vi "WHD_VEten_0.1_BIDIREC_Pruebas.vi"() -> ()   [LabVIEW 2015]
uses:
  <vilib>/NI_Real-Time Target Support.lvlib
  <vilib>/rvi/interface/nirviReadWriteControl/nirviReadWriteControl.xnode
  <vilib>/rvi/interface/nirviMethod/nirviMethod.xnode
  <vilib>/rvi/interface/nirviOpenFPGA/nirviOpenFPGA.xnode
  <vilib>/rvi/interface/nirviCloseFPGA/nirviCloseFPGA.xnode
  <vilib>/real-time/NI_Real-Time Libraries.lvlib
  <vilib>/userdefined/High Color/nirio_resource_hc.ctl
  <vilib>/Utility/file.llb/Write To Spreadsheet File (string).vi
  AURA_Wheel/Json2Labv.lvlib
  AURA_Wheel/AuraWheelAPI/AuraWheel.lvlib
  <vilib>/LabVIEW Targets/FPGA/cRIO/shared/nicrio_ModuleControls/nicrio_cRIO-9234_DataRatesRing2.ctl
  <vilib>/real-time/rtutility.llb/RT Restart Target (Self).vi
  FPGA Bitfiles/W&RDEuskotren_FPGATarget_FPGA8awsBIdirecc_10D55B35.lvbitx
  <vilib>/FPGAPlugInAG/cRIO-9113/niLvFpga_Open_cRIO-9113.vi
  <vilib>/FPGAPlugInAG/cRIO-9113/niLvFpga_Run_cRIO-9113.vi
  NiFpgaLv.dll
  <vilib>/Utility/error.llb/Error Cluster From Error Code.vi
  <vilib>/rvi/errors/niLvFpgaAdjustHostInterfaceError.vi
  <vilib>/FPGAPlugInAG/cRIO-9113/niLvFpga_ConfigureFifo_cRIO-9113.vi
  <vilib>/rvi/errors/niLvFpgaMergeErrorWithErrorCode.vi
  <vilib>/FPGAPlugInAG/cRIO-9113/niLvFpga_StartFifo_cRIO-9113.vi
  <vilib>/FPGAPlugInAG/cRIO-9113/niLvFpga_ReadFifo_cRIO-9113.vi
  <vilib>/FPGAPlugInAG/cRIO-9113/niLvFpga_StopFifo_cRIO-9113.vi
  <vilib>/FPGAPlugInAG/cRIO-9113/niLvFpga_Reset_cRIO-9113.vi
  <vilib>/FPGAPlugInAG/cRIO-9113/niLvFpga_Close_cRIO-9113.vi
  <vilib>/RTwatchdog.llb/Watchdog expiration actions.ctl
panel:
  out "TAGs_AURAwheel":string[][](array[string])
  out "Plataformas?":bool
  out "Ejes_convoy":i32
  out "Nº Ejes":i32[](array[numeric])
  out "Nº UTs":i32
  out "it-read-LR6":i32[](array[numeric])
  out "it-LR6":i32
  out "RFID_LR6_Error":errorcluster
  out "TAGs HEX":string[](array[string])
  out "TAGs LR6":string[](array[string])
  in  "TAGs HEX 2":string[](array[string])
  out "Series_flota":string[](array[string])
  out "Tabla_flota":string[][](array[string])
  out "Puntos medios de las ventanas":dbl[][](array[numeric])
  in  "User":string
  in  "Índice de los archivos seleccionados":i32
  in  "Array":path[][](array[path])=[[path "c:/Trenes_prueba/0207_2013-09-24_19-09-42_0.bin", path "c:/Trenes_prueba/0096_2013-10-30_18-13-14_0.bin", path "c:/Trenes_prueba/0001_2013-06-05_13-06-23_0.bin"], [path "c:/Trenes_prueba/0207_2013-09-24_19-09-42_1.bin", path "c:/Trenes_prueba/0096_2013-10-30_18-13-14_1.bin", path "c:/Trenes_prueba/0001_2013-06-05_13-06-23_1.bin"], [path "c:/Trenes_prueba/0207_2013-09-24_19-09-42_2.bin", path "c:/Trenes_prueba/0096_2013-10-30_18-13-14_2.bin", path "c:/Trenes_prueba/0001_2013-06-05_13-06-23_2.bin"], [path "c:/Trenes_prueba/0207_2013-09-24_19-09-42_3.bin", path "c:/Trenes_prueba/0096_2013-10-30_18-13-14_3.bin", path "c:/Trenes_prueba/0001_2013-06-05_13-06-23_3.bin"], [path "c:/Trenes_prueba/0207_2013-09-24_19-09-42_4.bin", path "c:/Trenes_prueba/0096_2013-10-30_18-13-14_4.bin", path "c:/Trenes_prueba/0001_2013-06-05_13-06-23_4.bin"], [path "c:/Trenes_prueba/0207_2013-09-24_19-09-42_5.bin", path "c:/Trenes_prueba/0096_2013-10-30_18-13-14_5.bin", path "c:/Trenes_prueba/0001_2013-06-05_13-06-23_5.bin"], [path "c:/Trenes_prueba/0207_2013-09-24_19-09-42_6.bin", path "c:/Trenes_prueba/0096_2013-10-30_18-13-14_6.bin", path "c:/Trenes_prueba/0001_2013-06-05_13-06-23_6.bin"], [path "c:/Trenes_prueba/0207_2013-09-24_19-09-42_7.bin", path "c:/Trenes_prueba/0096_2013-10-30_18-13-14_7.bin", path "c:/Trenes_prueba/0001_2013-06-05_13-06-23_7.bin"], [path "c:/Trenes_prueba/0207_2013-09-24_19-09-42_8.bin", path "c:/Trenes_prueba/0096_2013-10-30_18-13-14_8.bin", path "c:/Trenes_prueba/0001_2013-06-05_13-06-23_8.bin"]]
  out "configuration file path":path=path "c:/Parametros.cfg"
  in  "IP synchr":string
  in  "Canal ccero?":bool
  in  "Digital?":bool=TRUE
  out "Numeric 3":i32
  out "data":cluster{"status":string}
  out "confRFID":path=path "c:/RFID/TAGS.csv"
  out "TAGS leidos":path=path "c:/RFID/TAGS.csv"
  in  "Use Aura?":bool
  in  "Parametros AuraWheel":string[](array[string])
  in  "Parámetros acelerómetros":dbl[](array[numeric])
  in  "Number of Samples":u32=2000
  in  "x*y":dbl[](array[numeric])=array[252000 elements]
  out "RFID_Error 2":errorcluster
  in  "milliseconds to wait":u32=180000
  in  "Adquirir continuado":bool
  in  "Tiempo de adquisicion":dbl=10.0
  in  "Adquirir":bool
  in  "Señal digital?":bool=TRUE
  out "Inductivo OK?":bool=TRUE
  out "Acelerómetros OK?":bool[](array[boolean])
  out "Fin":bool
  out "Contador":i32=1
  in  "expiration actions":T1={"reset"=TRUE, "occurrence"=FALSE, "trigger protocol"=enum."active high", "trigger line"=enum."none", "disable watchdog on VI exit"=TRUE}
  out "Path TEST":path=path "c:/TEST"
  out "Fallo fotocelula":bool
  out "Path_Borrar":path=path "c:/Trenes"
  out "Longitud de la unidad":dbl
  out "Bucle Espera":i32
  out "Aviso no detección":string
  out "Time to Acquire Block (ms)":i32
  out "Distancia de acelerómetros":dbl[](array[numeric])
  out "Block Size":u32
  out "Distancias generales":dbl[](array[numeric])
  in  "Reset del controlador":bool
  in  "Configuración":bool
  in  "Parar la aplicación":bool
  out "Acel 4":bool=TRUE
  out "Acel 3":bool=TRUE
  out "Acel 2":bool=TRUE
  out "Acel 1":bool=TRUE
  out "RFID":bool=TRUE
  out "date/time string":string
  out "Obstruido?":bool
  out "Tiempo":dbl
  out "Inicio pasada":timestamp
  out "Ultimo TEST":timestamp
  out "Fuente":bool=TRUE
  out "Estado":string
  in  "Number of Channels":u32=9
  out "RFID_ID":refnum<k5>
  out "DC OK":string
  out "Aviso temperatura":string
  in  "Tab Control":T2(tab)=enum."Parámetros"
  out "V (m/s)":dbl
  out "Temperatura (ºC)":dbl
  out "Max RMS Ruedas":dbl[][](array[numeric])
  in  "Hora de borrado":string
  out "result":bool
  out "TAGs":string[](array[string])
  out "Nombre de archivo":path[](array[path])
  out "Tiempo de paso (s)":dbl
  out "Tiempo extra de adquisición (s)":dbl
  out "Número de ejes detectados":i32
  out "Buffer Underflow":bool
  out "Buffer Overflow":bool
  out "Disco Duro Disponible (bytes)":i64
  out "created path":path
  out "Fallo sensores":string
  out "T fuera rango":bool
  in  "Frecuencia de muestreo (Hz)":dbl=25600.0
  in  "Escaneos de la FIFO por canal":u32=1000
  in  "Tiempo extra al detector de paso (s)":dbl=1.0
  in  "Filtro digital (ms)":u16=13
  in  "dt RMS":dbl=256.0
  in  "Time":T3 {"Segundo" min=0 max=60; "Minuto" min=0 max=60; "Hora" min=0 max=24}
  in  "Cambiar hora":bool
  in  "Date":T4={"Mes   "=1, "Día         "=1, "Año "=2010} {"Año" min=1900 max=3000 step=1; "Día" min=1 max=31 step=1; "Mes" min=1 max=12 step=1}
  in  "Cambiar Fecha":bool
  in  "Frecuencia de muestreo y módulo CRIO":T5=2 items=["51.200 kS/s (NI 9234)"=1, "25.600 kS/s (NI 9234)"=2, "17.067 kS/s (NI 9234)"=3, "12.800 kS/s (NI 9234)"=4, "10.240 kS/s (NI 9234)"=5, "8.533 kS/s (NI 9234)"=6, "7.314 kS/s (NI 9234)"=7, "6.400 kS/s (NI 9234)"=8, "5.689 kS/s (NI 9234)"=9, "5.120 kS/s (NI 9234)"=10, "4.654 kS/s (NI 9234)"=11, "4.267 kS/s (NI 9234)"=12, "3.938 kS/s (NI 9234)"=13, "3.657 kS/s (NI 9234)"=14, "3.413 kS/s (NI 9234)"=15, "3.200 kS/s (NI 9234)"=16, "3.012 kS/s (NI 9234)"=17, "2.845 kS/s (NI 9234)"=18, "2.695 kS/s (NI 9234)"=19, "2.560 kS/s (NI 9234)"=20, "2.438 kS/s (NI 9234)"=21, "2.328 kS/s (NI 9234)"=22, "2.226 kS/s (NI 9234)"=23, "2.133 kS/s (NI 9234)"=24, "2.048 kS/s (NI 9234)"=25, "1.969 kS/s (NI 9234)"=26, "1.896 kS/s (NI 9234)"=27, "1.829 kS/s (NI 9234)"=28, "1.765 kS/s (NI 9234)"=29, "1.707 kS/s (NI 9234)"=30, "1.652 kS/s (NI 9234)"=31]
  in  "Puerto RFID":u16=2189
  in  "IP RFID":string="192.168.106.99"
  in  "Offset_rueda":fxp<+/-,24,-4>=0.004999998956918716 format="%.27g"
  in  "Count(mSec)":u32=2
  in  "LR6 IP address":string="192.168.106.94"
  in  "Port LR6":u16=2001
  out "Direccion 0?":bool
  in  "Pruebas RFID 2":bool
  in  "Pruebas RFID 1":bool
  in  "Descargar":bool
  out "Parámetros":bool=TRUE
  out "Distacias y medidas de dispositivos":bool=TRUE
  out "RFID_Error":errorcluster
  out "error FPGA":errorcluster
  out "error manipulacion archivos":errorcluster
  out "Unidades y ejes":bool=TRUE
  out "RFID":bool=TRUE
  out "error AURA":errorcluster
  out "Response headers":string
  # "Funciona?"
  # "Inductivo"
  # "A4"
  # "A3"
  # "A1"
  # "A2"
  # "WRD_MEX\nWRD_ZAR"
  # "0 tagMexInit\n1 tagMexFin\n\n0 tag1\n1 tag2"
  # "Última detección de unidad"
  # "Error!!"
  # "Estado de la memoria"
  # "Espera"
  # "Adquisicion"
  # "Adquisicion"
  # "Procesado"
  # "Procesado"
  # "Procesado"
  # "Procesado"
  # "Procesado"
  # "Parámetros de muestreo"
  # "Parámetros de adquisición"
  # "Parámetros de procesado"
  # "Cambio Fecha y Hora"
  # "Descarga de planos y TEST"
  # "NO"
  # "SI"
  # "Descarga archivos binarios de adquisición"
  # "NO"
  # "SI"
  # "Cargar datos de configuración"
  # "Errores!!"
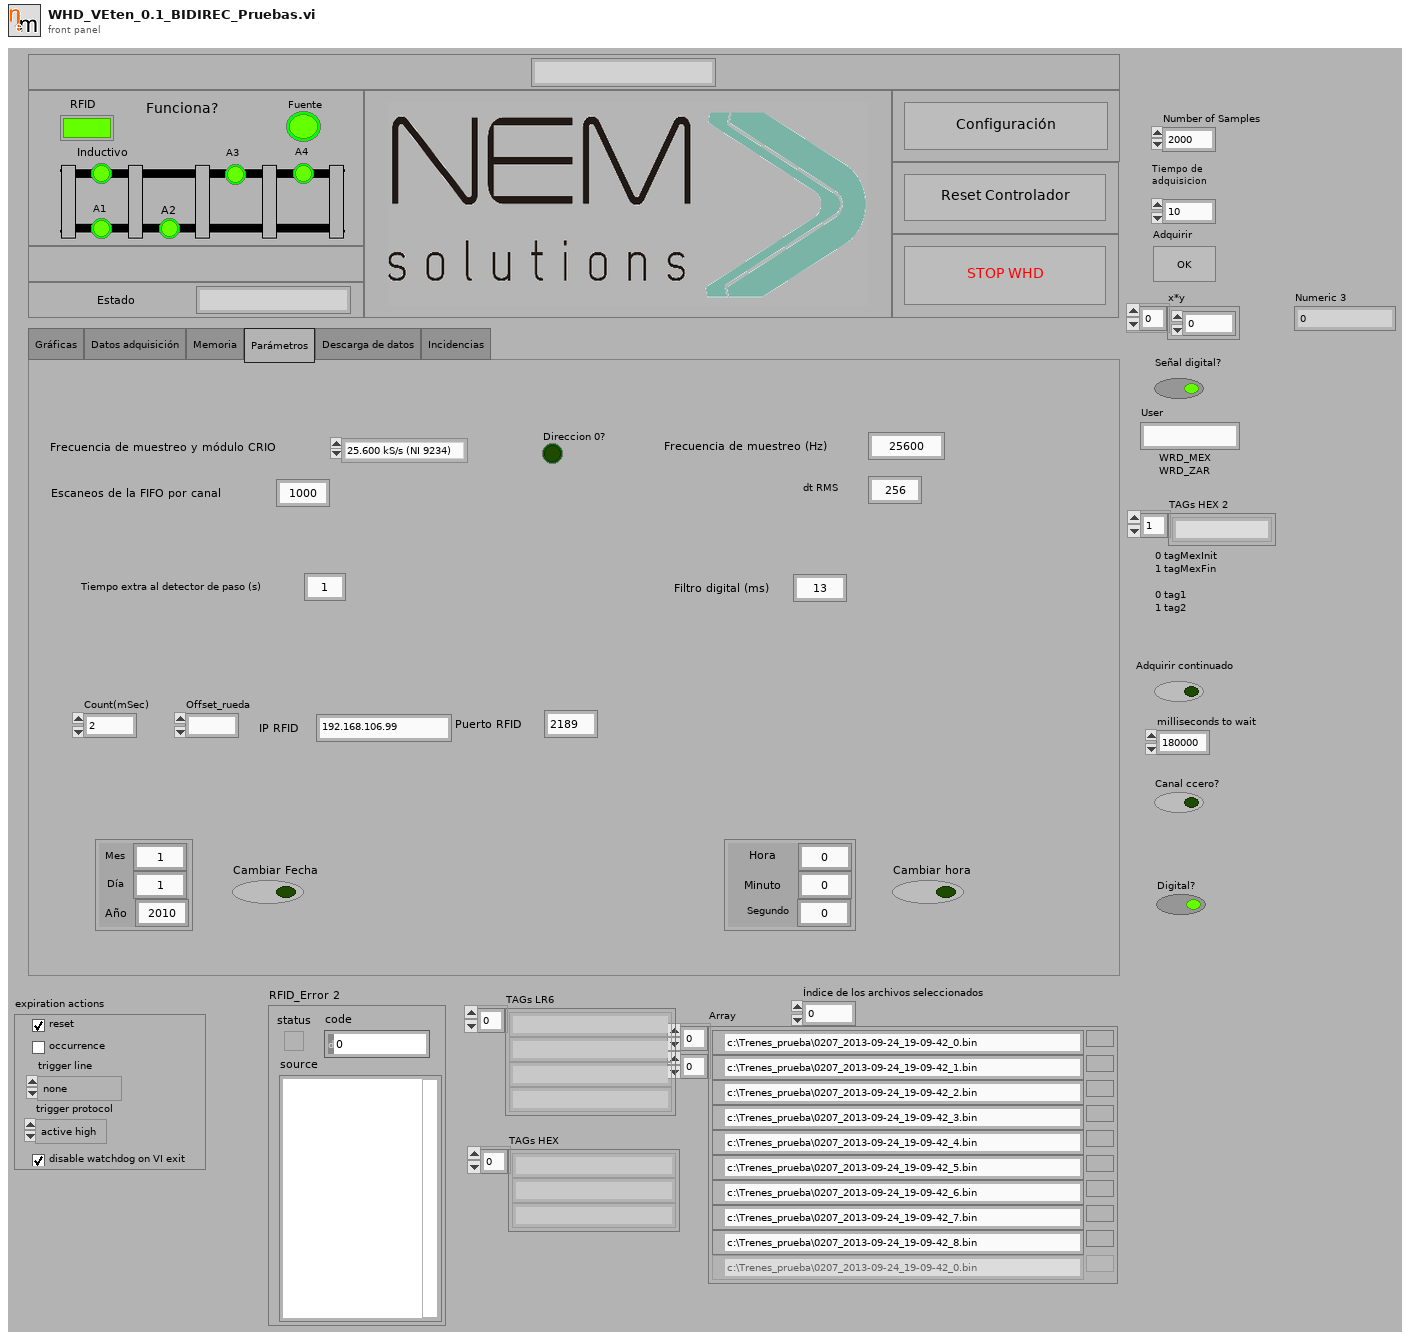
[diagram p1: front panel]
types:
  T1 = typedef "Watchdog expiration actions.ctl" = cluster{"reset":bool, "occurrence":bool, "trigger protocol":enum16{"active high", "active low", "open collector"}, "trigger line":enum16{"none", "line 0", "line 1", "line 2", "line 3", "line 4", "line 5", "line 6", "line 7", "SMB line 0"}, "disable watchdog on VI exit":bool}
  T2 = enum32{"Gráficas", "Datos adquisición", "Memoria", "Parámetros", "Descarga de datos", "Incidencias"}
  T3 = cluster{"Hora        ":i32, "Minuto     ":i32, "Segundo               ":i32}
  T4 = cluster{"Mes   ":i32, "Día         ":i32, "Año ":i32}
  T5 = typedef "nicrio_cRIO-9234_DataRatesRing2.ctl" = u8
  T6 = typedef "nirio_resource_hc.ctl" = tag
  T7 = enum16{"Standard", "Buffered", "CRLF", "Immediate"}
  T8 = enum16{"open", "replace", "create", "open or create", "replace or create", "replace or create with confirmation"}
  T9 = enum16{"big-endian, network order", "native, host order", "little-endian"}
  T10 = cluster{"error IO":errorcluster, bool[], u32[], string[], dbl[]}
  T11 = cluster{"g_ts":dbl, "p_sp":dbl, "p_tp":dbl, "p_tg":cluster{"tg_n":dbl, "tg_t":string}[], "p_ax":cluster{"ax_n":dbl, "ax_sp":dbl, "ax_wh":cluster{"wh_p":dbl, "wh_a1":dbl, "wh_a2":dbl, "wh_a3":dbl, "wh_a4":dbl}[]}[]}
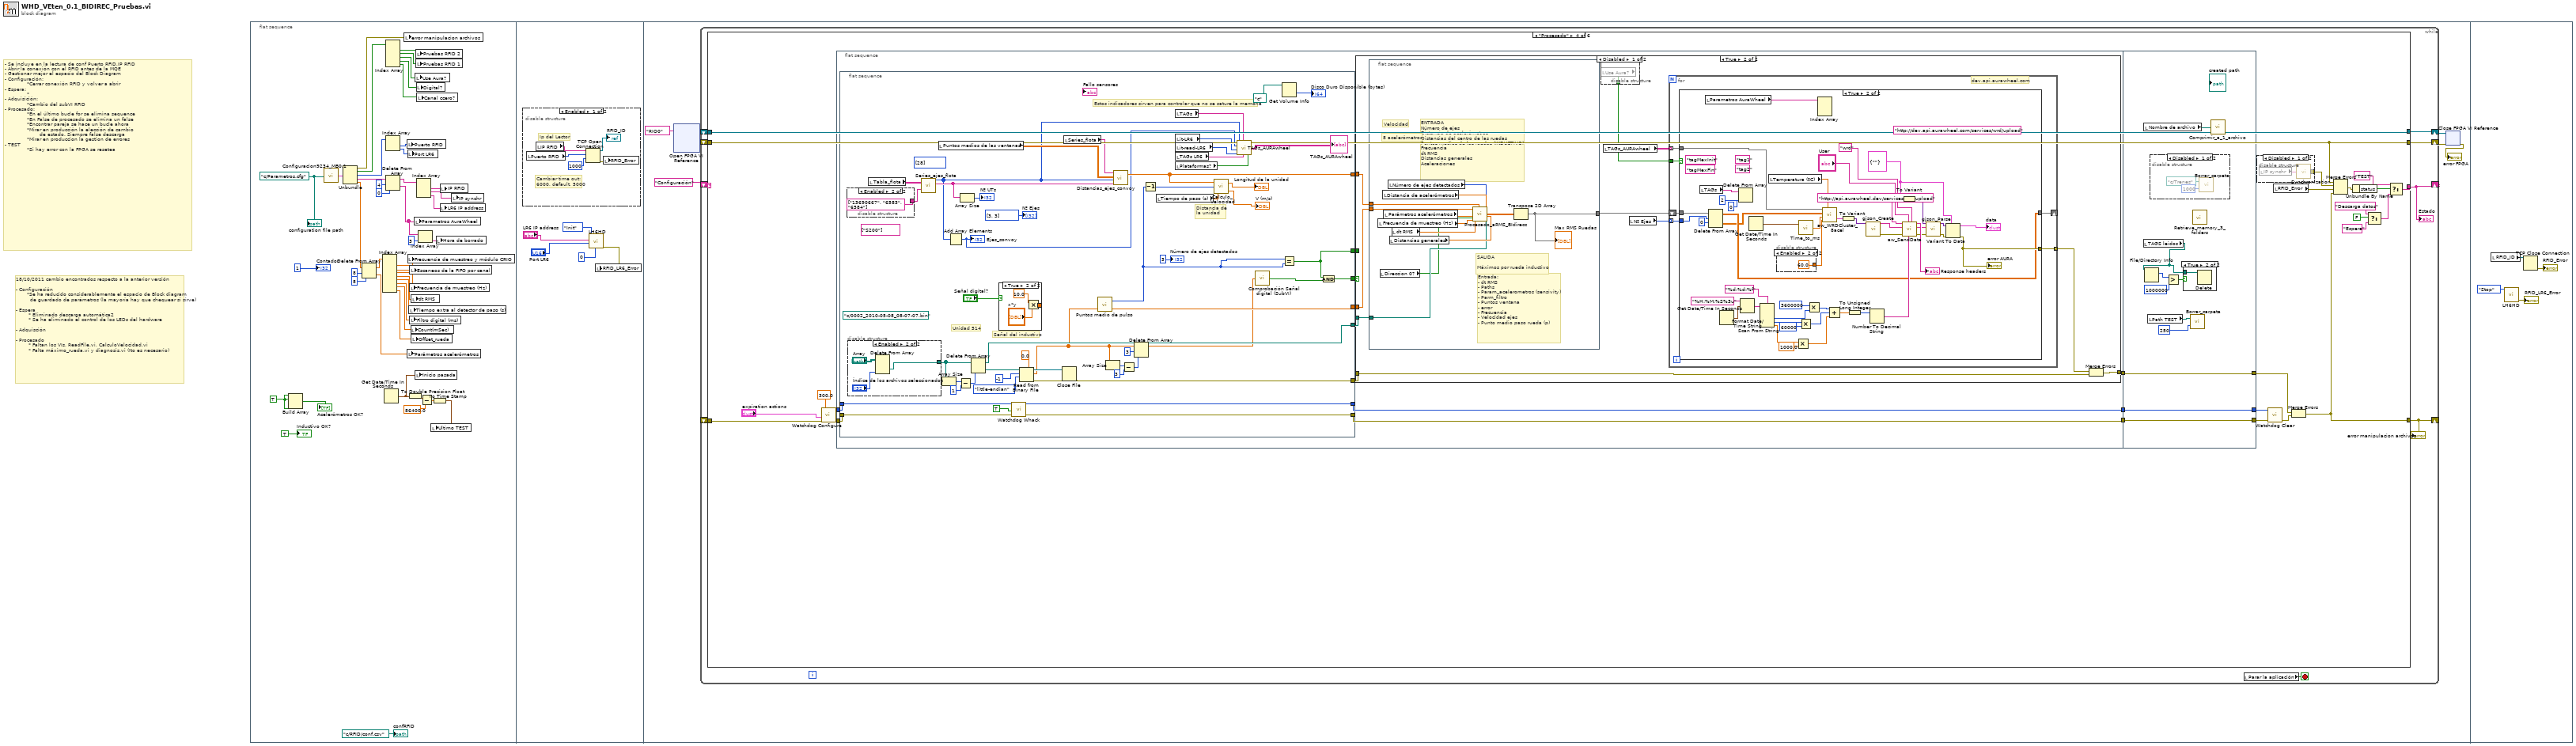
[diagram p0: block diagram]
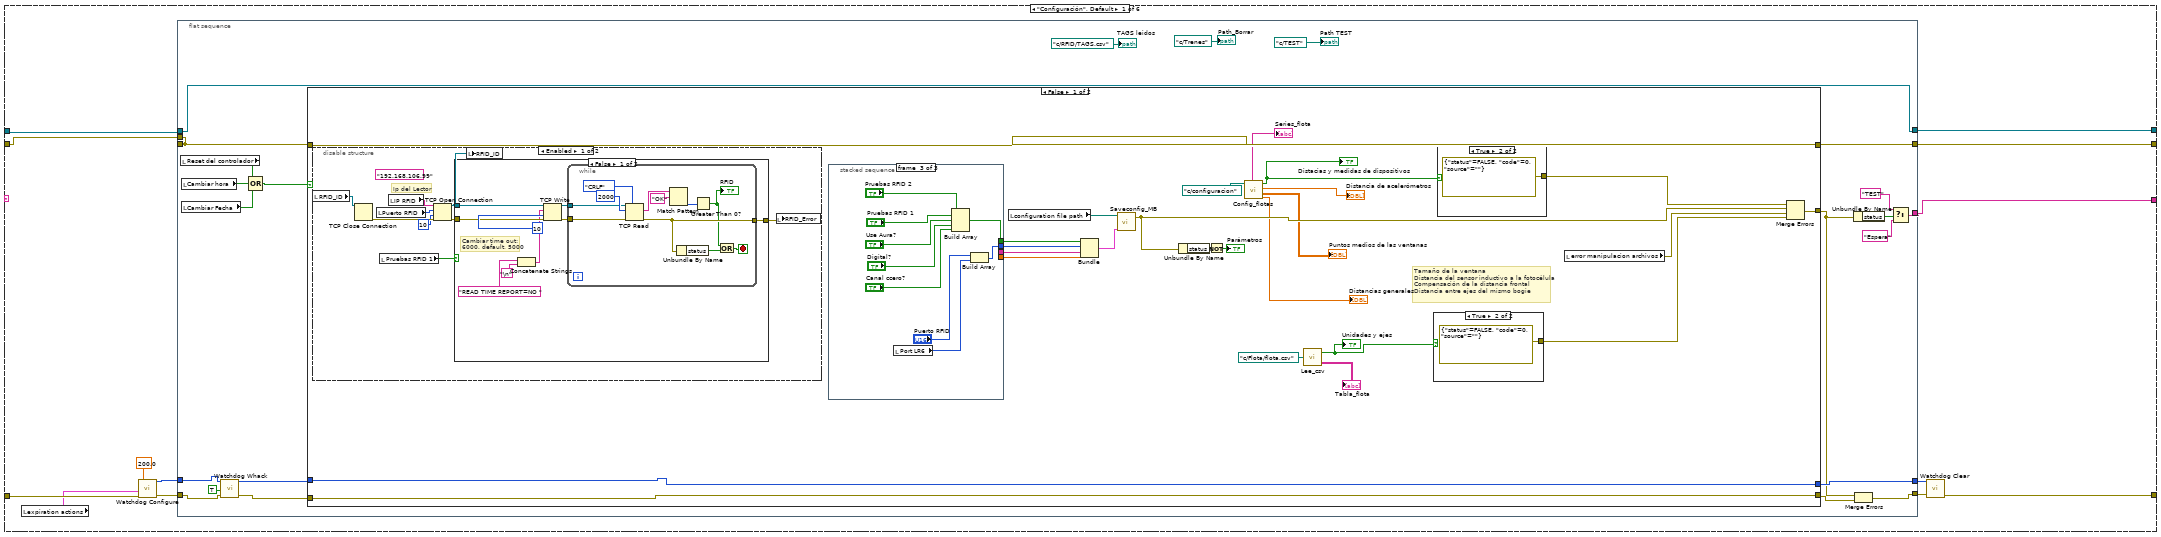
[diagram p3: hidden frame]
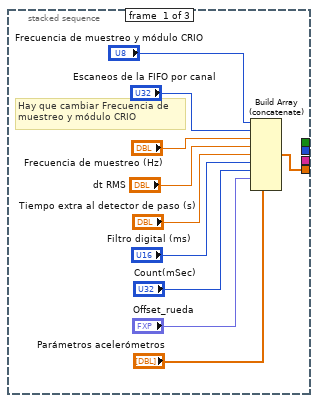
[diagram p4: hidden frame]
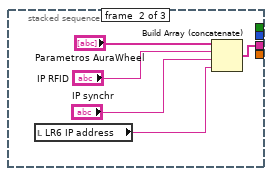
[diagram p5: hidden frame]
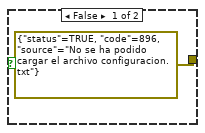
[diagram p6: hidden frame]
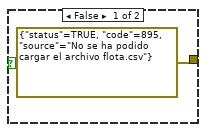
[diagram p7: hidden frame]
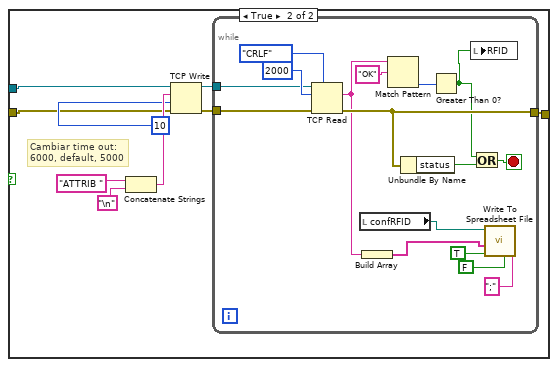
[diagram p8: hidden frame]
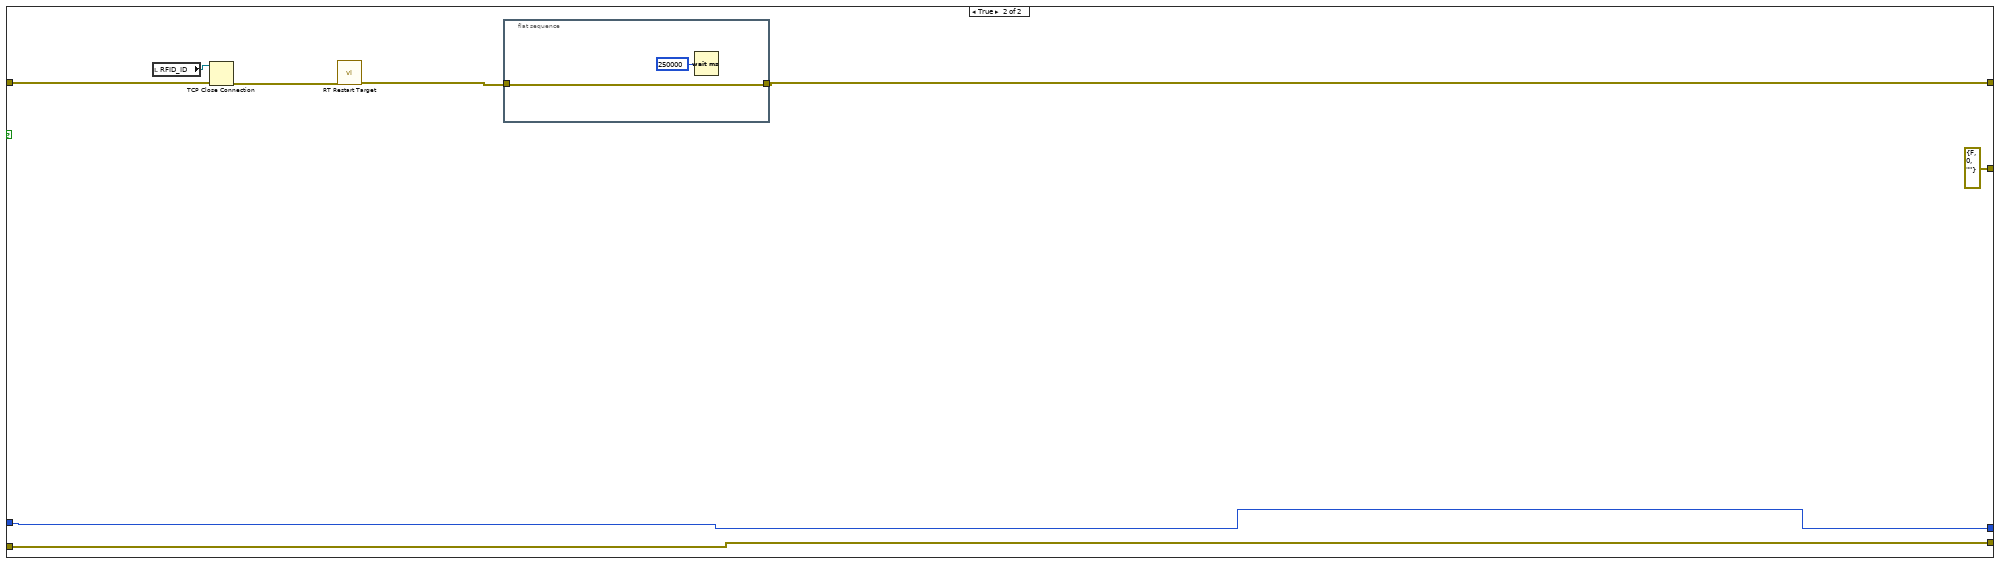
[diagram p10: hidden frame]
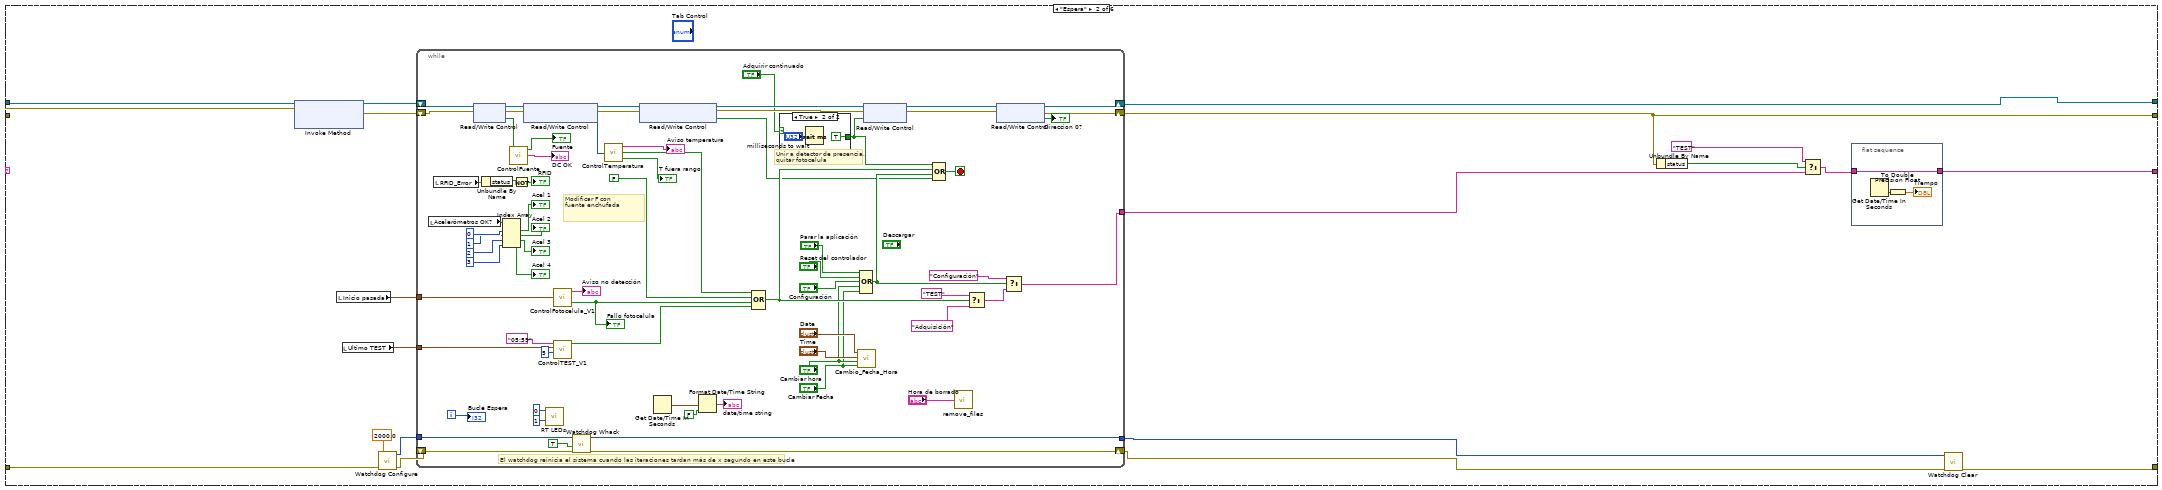
[diagram p11: hidden frame]
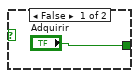
[diagram p12: hidden frame]
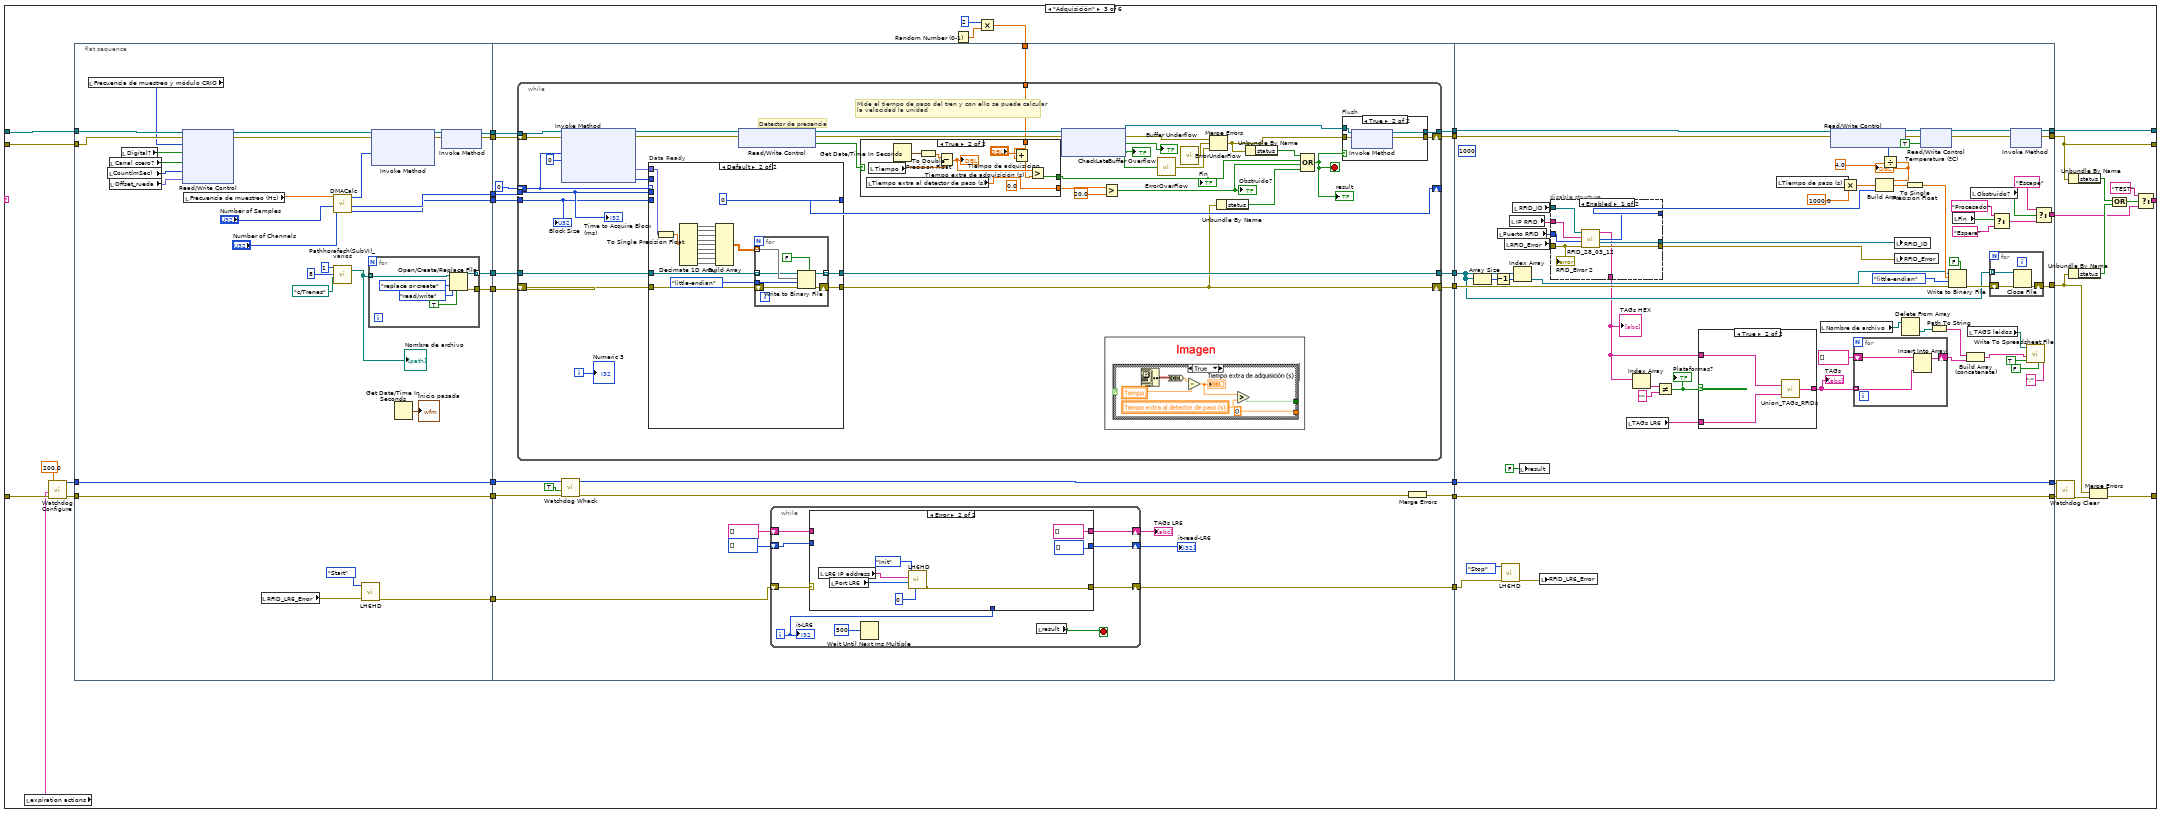
[diagram p13: hidden frame]
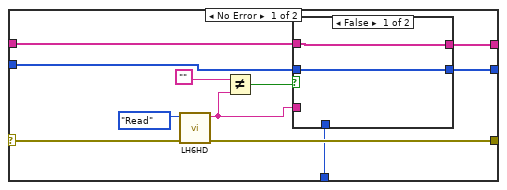
[diagram p14: hidden frame]
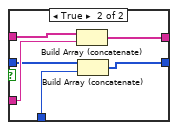
[diagram p15: hidden frame]
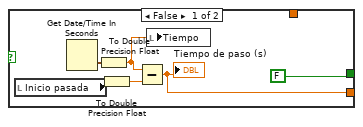
[diagram p16: hidden frame]
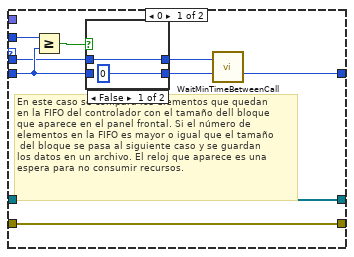
[diagram p17: hidden frame]
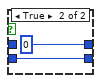
[diagram p18: hidden frame]
diagram:
  # "18/10/2011 cambio encontrados respecto a la anterior versión\n\n- Configuración\n       *Se ha reducido considerablemente el espacio de Block diagram\n         de guardado de parámetros (la mayoría hay que chequear si sirve)\n\n- Espera\n        * Eliminado descarga automática2\n        * Se ha eliminado el control de los LEDs del hardware\n       \n- Adquisción\n\n- Procesado\n        * Faltan los VIs, ReadFile.vi, CalculoVelocidad.vi\n        * Falta máximo_rueda.vi y diagnosis.vi (No es necesario)"
  # "- Se incluye en la lectura de conf Puerto RFID,IP RFID\n- Abrir la conexión con el RFID antes de la MQE\n- Gestionar mejor el espacio del Block Diagram\n- Configuración:\n              *Cerrar conexión RFID y volver a abrir\n- Espera:\n              *\n- Adquisición:\n              *Cambio del subVI RFID\n- Procesado:\n              *En el último bucle for se elimina sequence\n              *En False de procesado se elimina un false\n              *Encontrar pareja se hace un bucle ahora\n              *Mirar en producción la elección de cambio\n                      de estado. Siempre false descarga \n              *Mirar en produccion la gestion de errores\n- TEST\n              *Si hay error con la FPGA se resetea"
  n1 = flat-sequence {
    frame #0 {
      w29 = TRUE
      w25 = path "c:/Parametros.cfg" ("configuration file path")
      n2 = Build Array(w29, w29, w29, w29) -> (→"Acelerómetros OK?":bool[])
      n3 = call "Configuracion9234_MB0.1.vi"("configuration file path"=w25) -> ("output cluster"=w24:T10)
      n4 = Unbundle(w24) -> ("error IO"=w32:errorcluster, w31:bool[], w30:u32[], w16:string[], w22:dbl[])
      n5 = Delete From Array(array=w22, length=8, index=8) -> (deleted portion=w18:dbl[], array with subset deleted=w21:dbl[])
      n6 = Index Array(array=w21) -> (element #1=w40:dbl, element #2=w39:dbl, element #3=w38:dbl, element #4=w37:dbl, element #5=w36:dbl, element #6=w35:dbl, element #7=w8:dbl, element #8=w7:dbl)  [unwired: 8 in]
      n7 = Get Date/Time In Seconds() -> (seconds since 1Jan1904=w42:timestamp)
      n8 = Index Array(array=w31) -> (element #1=w34:bool, element #2=w33:bool, element #3=w17:bool, element #4=w4:bool, element #5=w9:bool)  [unwired: 5 in]
      n9 = Index Array(array=w30) -> (element #1=w23:u32, element #2=w1:u32)  [unwired: 2 in]
      n10 = Delete From Array(array=w16, length=4, index=0) -> (deleted portion=w5:string[], array with subset deleted=w15:string[])
      n11 = local write "error manipulacion archivos"(w32) -> ()
      n12 = local write "Puerto RFID"(w23) -> ()
      n13 = local write "Parámetros acelerómetros"(w18) -> ()
      n14 = local write "Port LR6"(w1) -> ()
      n15 = local write "Frecuencia de muestreo y módulo CRIO"(w40) -> ()
      n16 = To Double Precision Float(number=w42) -> (double precision float=w44:dbl)
      n17 = local write "Tiempo extra al detector de paso (s)"(w36) -> ()
      n18 = local write "Frecuencia de muestreo (Hz)"(w38) -> ()
      n19 = local write "Filtro digital (ms)"(w35) -> ()
      n20 = local write "Escaneos de la FIFO por canal"(w39) -> ()
      n21 = local write "Count(mSec)"(w8) -> ()
      n22 = local write "dt RMS"(w37) -> ()
      n23 = local write "Offset_rueda"(w7) -> ()
      n24 = local write "Parametros AuraWheel"(w5) -> ()
      n25 = local write "Inicio pasada"(w42) -> ()
      n26 = local write "Use Aura?"(w17) -> ()
      n27 = local write "Pruebas RFID 2"(w34) -> ()
      n28 = local write "Pruebas RFID 1"(w33) -> ()
      n29 = local write "Digital?"(w4) -> ()
      n30 = Index Array(array=w15) -> (element #1=w3:string, element #2=w6:string, element #3=w2:string)  [unwired: 3 in]
      n31 = local write "Canal ccero?"(w9) -> ()
      n32 = Index Array(array=w5, index=3) -> (element=w10:string)
      n33 = Subtract(x=w44, y=86400.0) -> (x-y=w43:dbl)
      n34 = To Time Stamp(1:w43) -> (0:w41:timestamp)
      n35 = local write "Ultimo TEST"(w41) -> ()
      n36 = local write "Hora de borrado"(w10) -> ()
      n37 = local write "IP RFID"(w3) -> ()
      n38 = local write "LR6 IP address"(w2) -> ()
      n39 = local write "IP synchr"(w6) -> ()
      "Contador" <- 1
      "Inductivo OK?" <- TRUE ("Inductivo OK?")
      "confRFID" <- path "c:/RFID/conf.csv" ("file path (use dialog)")
      "configuration file path" <- w25
    }
    frame #1 {
      n40 = disable-structure shown="Enabled" {
        frame Enabled {
          # "Cambiar time out:\n6000, default, 5000"
          # "Ip del Lector"
          n41 = local read "Puerto RFID"() -> (w52:u16)
          n42 = local read "IP RFID"() -> (w53:string)
          n43 = TCP Open Connection(address=w53, remote port or service name=w52, timeout ms (60000)=1000) -> (connection ID=→"RFID_ID":refnum<k5>, error out=w51:errorcluster)  [unwired: 1 in, 1 out]
          n44 = local write "RFID_Error"(w51) -> ()
        }
        frame Disabled {
        }
      }
      n45 = call "LH6HD.vi"("DeviceAddress"=u8 0, "Reader Port"="Port LR6", "IP Address"="LR6 IP address", "Action"=enum16{"Init", "Start", "Read", "Stop", "Exit"}."Init") -> ("error out"=w46:errorcluster)  [unwired: 6 in, 1 out]
      n46 = local write "RFID_LR6_Error"(w46) -> ()
    }
    frame #2 {
      n47 = xnode "Open FPGA VI Reference"("resource name"=T6 "RIO0") -> ("FPGA VI Reference Out"=w62:refnum<k20>, "error out"=w61:errorcluster)  [unwired: 1 in]
      n48 = while {
        shift-right: [w66] -> _
        shift-left: "Configuración" -> [w71]
        shift-right: [w64] -> w58
        shift-left: w62 -> [w70]
        shift-right: [w63] -> w57
        shift-left: w61 -> [w69]
        shift-right: [w68] -> _
        shift-left: _ -> [w67]
        stop <- w65 stop-if-true
        n49 = case shown="\"Procesado\"" w71 {
          tunnel: [w83 w228 w327 w641 w862 "TEST" ("t")] -> w66
          tunnel: [w82 w227 w348 w656 w860 w929] -> w64
          tunnel: [w84 w225 w349 w633 w851 w926] -> w63
          tunnel: w70 -> [w73 w234 w359 w656 w860 w928]
          tunnel: w69 -> [w72 w232 w358 w633 w859 w925]
          tunnel: [w75 w226 w344 w638 w858 w930] -> w68
          tunnel: w67 -> [w80 w242 w350 w654 w861 w930]
          frame "Configuración", Default {
            n50 = local read "expiration actions"() -> (w74:T1)
            n51 = call <vilib>:"Watchdog Configure.vi"("error in (no error)"=w80, "expiration actions"=w74, "timeout (1 sec)"=200.0) -> ("error out"=w79:errorcluster, "watchdogID"=w78:u64)  [unwired: 3 out]
            n52 = flat-sequence {
              tunnel: [w85] -> _
              tunnel: [w94] -> w84
              tunnel: [w106] -> w83
              tunnel: w73 -> [w95]
              tunnel: [w95] -> w82
              tunnel: w79 -> [w89]
              tunnel: w78 -> [w87]
              tunnel: [w93] -> w77
              tunnel: [w97] -> w76
              tunnel: w72 -> [w85]
              frame #0 {
                n53 = local read "Reset del controlador"() -> (w102:bool)
                n54 = local read "Cambiar hora"() -> (w101:bool)
                n55 = local read "Cambiar Fecha"() -> (w100:bool)
                n56 = call <vilib>:"Watchdog Whack.vi"("error in (no error)"=w89, "reset watchdog after expire? (F)"=TRUE, "watchdogID in"=w87) -> ("error out"=w88:errorcluster, "watchdogID out"=w86:u64)  [unwired: 3 out]
                n57 = Compound Arithmetic op=OR(w102, w101, w100) -> (w99:bool)
                n58 = case shown="False" w99 {
                  tunnel: w85 -> [w132 w220]
                  tunnel: [w132 w217] -> w94
                  tunnel: [w118 errorcluster {"status"=FALSE, "code"=0, "source"=""} ("error IO")] -> w92
                  tunnel: w86 -> [w117 w216]
                  tunnel: w88 -> [w116 w215]
                  tunnel: [w117 w216] -> w93
                  tunnel: [w116 w215] -> w91
                  frame False {
                    # "Tamaño de la ventana\nDistancia del sensor inductivo a la fotocélula\nCompensación de la distancia frontal\nDistancia entre ejes del mismo bogie"
                    n59 = disable-structure shown="Enabled" {
                      frame Enabled {
                        (unwired) "192.168.106.99" ("address")
                        # "Ip del Lector"
                        n60 = local read "RFID_ID"() -> (w168:refnum<k5>)
                        n61 = TCP Close Connection(connection ID=w168) -> (error out=w169:errorcluster)  [unwired: 2 in, 1 out]
                        n62 = local read "Puerto RFID"() -> (w166:u16)
                        n63 = local read "Pruebas RFID 1"() -> (w161:bool)
                        n64 = local read "IP RFID"() -> (w165:string)
                        n65 = TCP Open Connection(address=w165, remote port or service name=w166, timeout ms (60000)=10, error in (no error)=w169) -> (connection ID=w167:refnum<k5>, error out=w162:errorcluster)  [unwired: 1 out]
                        n66 = case shown="False" w161 {
                          tunnel: w167 -> [w178 w192]
                          tunnel: [w176 w190] -> w163
                          tunnel: w162 -> [w173 w191]
                          frame False {
                            # "Cambiar time out:\n6000, default, 5000"
                            n67 = Concatenate Strings("READ TIME REPORT=NO " ("data in"), "\n") -> (w170:string)
                            n68 = TCP Write(connection ID=w178, data in=w170, error in (no error)=w173, 9:10 ("timeout ms (25000)")) -> (connection ID out=w174:refnum<k5>, error out=w175:errorcluster)  [unwired: 1 out]
                            n69 = while {
                              tunnel: w175 -> [w187]
                              tunnel: w174 -> [w186]
                              tunnel: [w185] -> w176
                              stop <- w182 stop-if-true
                              n70 = TCP Read(connection ID=w186, bytes to read=2000, error in (no error)=w187, 7:T7."CRLF" ("mode (standard)")) -> (data out=w180:string, error out=w185:errorcluster)  [unwired: 1 in, 1 out]
                              n71 = Match Pattern(string=w180, regular expression="OK") -> (offset past match=w183:i32)  [unwired: 4 out]
                              n72 = Unbundle By Name(w185) -> ("status"=w181:bool)
                              n73 = Greater Than 0?(x=w183) -> (x > 0?=w179:bool)
                              "RFID" <- w179
                              n74 = Or(x=w179, y=w181) -> (x .or. y?=w182:bool)
                            }
                          }
                          frame True {
                            # "Cambiar time out:\n6000, default, 5000"
                            n75 = Concatenate Strings("ATTRIB " ("data in"), "\n") -> (w198:string)
                            n76 = TCP Write(connection ID=w192, data in=w198, error in (no error)=w191, 9:10 ("timeout ms (25000)")) -> (connection ID out=w195:refnum<k5>, error out=w194:errorcluster)  [unwired: 1 out]
                            n77 = while {
                              tunnel: w194 -> [w212]
                              tunnel: w195 -> [w211]
                              tunnel: [w210] -> w190
                              stop <- w207 stop-if-true
                              n78 = TCP Read(connection ID=w211, bytes to read=2000, error in (no error)=w212, 7:T7."CRLF" ("mode (standard)")) -> (data out=w201:string, error out=w210:errorcluster)  [unwired: 1 in, 1 out]
                              n79 = local read "confRFID"() -> (w199:path)
                              n80 = Build Array(w201) -> (w200:string[])
                              n81 = Match Pattern(string=w201, regular expression="OK") -> (offset past match=w208:i32)  [unwired: 4 out]
                              n82 = Unbundle By Name(w210) -> ("status"=w206:bool)
                              n83 = Greater Than 0?(x=w208) -> (x > 0?=w205:bool)
                              n84 = local write "RFID"(w205) -> ()
                              n85 = Or(x=w205, y=w206) -> (x .or. y?=w207:bool)
                              n86 = call-poly <vilib>:"Write To Spreadsheet File.vi"("delimiter (\\t)"=";" ("delimiter (\\t)"), "transpose? (no:F)"=FALSE, "append to file? (new file:F)"=TRUE, "1D data"=w200, "file path (dialog if empty)"=w199) -> ()  [unwired: 3 in, 1 out]
                            }
                          }
                        }
                        n87 = local write "RFID_ID"(w167) -> ()
                        n88 = local write "RFID_Error"(w163) -> ()
                      }
                      frame Disabled {
                      }
                    }
                    n89 = stacked-sequence {
                      tunnel: [w137 _ _] -> w122
                      tunnel: [_ w147 _] -> w121
                      tunnel: [_ _ w153] -> w123
                      tunnel: [_ _ w152] -> w124
                      frame #0 {
                        # "Hay que cambiar Frecuencia de\nmuestreo y módulo CRIO"
                        n90 = Build Array (concatenate)("Frecuencia de muestreo y módulo CRIO", "Escaneos de la FIFO por canal", "Frecuencia de muestreo (Hz)", "dt RMS", "Tiempo extra al detector de paso (s)", "Filtro digital (ms)", "Count(mSec)", "Offset_rueda", "Parámetros acelerómetros") -> (w137:dbl[])
                      }
                      frame #1 {
                        n91 = local read "LR6 IP address"() -> (w143:string)
                        n92 = Build Array (concatenate)("Parametros AuraWheel", "IP RFID", "IP synchr", w143) -> (w147:string[])
                      }
                      frame #2 {
                        n93 = local read "Port LR6"() -> (w148:u16)
                        n94 = Build Array("Pruebas RFID 2", "Pruebas RFID 1", "Use Aura?", "Digital?", "Canal ccero?") -> (w152:bool[])
                        n95 = Build Array("Puerto RFID", w148) -> (w153:u16[])
                      }
                    }
                    n96 = local read "configuration file path"() -> (w119:path)
                    n97 = Bundle(w124, w123, w121, w122) -> (w120:cluster{bool[], u16[], string[], dbl[]})  [unwired: 1 in]
                    n98 = call "Saveconfig_MB.vi"("configuration file path"=w119, "Configuracion"=w120) -> ("error out"=w127:errorcluster)  [unwired: 4 in]
                    n99 = Unbundle By Name(w127) -> ("status"=w128:bool)
                    n100 = Not(x=w128) -> (.not. x?=→"Parámetros":bool)
                    n101 = call "Config_flotas.vi"("file path (dialog if empty)"=path "c:/configuracion") -> ("Distancias generales"=→"Distancias generales":dbl[], "Puntos medios de las ventanas"=→"Puntos medios de las ventanas":dbl[][], "Distancia de acelerómetros"=→"Distancia de acelerómetros":dbl[], "Distacias y medidas de dispositivos"=w115:bool, "Series_flota"=→"Series_flota":string[])  [unwired: 3 in]
                    "Distacias y medidas de dispositivos" <- w115
                    n102 = call "Lee_csv.vi"("Path"=path "c:/Flota/flota.csv") -> ("Tabla_flota"=→"Tabla_flota":string[][], "Lectura_OK?"=w111:bool)
                    "Unidades y ejes" <- w111
                    n103 = case shown="True" w111 {
                      tunnel: [errorcluster {"status"=TRUE, "code"=895, "source"="No se ha podido cargar el archivo flota.csv"} ("error out") errorcluster {"status"=FALSE, "code"=0, "source"=""} ("error out")] -> w125
                      frame False {
                      }
                      frame True {
                      }
                    }
                    n104 = case shown="True" w115 {
                      tunnel: [errorcluster {"status"=TRUE, "code"=896, "source"="No se ha podido cargar el archivo configuracion.txt"} ("error out") errorcluster {"status"=FALSE, "code"=0, "source"=""} ("error out")] -> w130
                      frame False {
                      }
                      frame True {
                      }
                    }
                    n105 = local read "error manipulacion archivos"() -> (w126:errorcluster)
                    n106 = Merge Errors(w130, w127, w126, w125) -> (w118:errorcluster)
                  }
                  frame True {
                    n107 = local read "RFID_ID"() -> (w222:refnum<k5>)
                    n108 = TCP Close Connection(connection ID=w222, error in (no error)=w220) -> (error out=w219:errorcluster)  [unwired: 2 out]
                    n109 = call-poly <vilib>:"RT Restart Target.vi"("error in (no error)"=w219) -> ("error out"=w218:errorcluster)  [unwired: 10 in]
                    n110 = flat-sequence {
                      tunnel: [w224] -> w217
                      tunnel: w218 -> [w224]
                      frame #0 {
                        n111 = Wait (ms)(milliseconds to wait=u32 250000) -> ()  [unwired: 1 out]
                      }
                    }
                  }
                }
                n112 = Unbundle By Name(w92) -> ("status"=w107:bool)
                n113 = Merge Errors(w92, w91) -> (w97:errorcluster)
                n114 = Select(t="TEST", s=w107, f="Espera") -> (s? t:f=w106:string)
                "Path_Borrar" <- path "c:/Trenes" ("file path (use dialog)")
                "Path TEST" <- path "c:/TEST" ("file path (use dialog)")
                "TAGS leidos" <- path "c:/RFID/TAGS.csv" ("file path (use dialog)")
              }
            }
            n115 = call <vilib>:"Watchdog Clear.vi"("error in (no error)"=w76, "watchdogID in"=w77) -> ("error out"=w75:errorcluster)  [unwired: 5 out]
          }
          frame "Espera" {
            n116 = xnode "Invoke Method"("FPGA VI Reference In"=w234, "error in"=w232) -> ("FPGA VI Reference Out"=w233:refnum<k20>, "error out"=w231:errorcluster)  [unwired: 1 in]
            n117 = local read "Inicio pasada"() -> (w239:timestamp)
            n118 = local read "Ultimo TEST"() -> (w238:timestamp)
            n119 = call <vilib>:"Watchdog Configure.vi"("error in (no error)"=w242, "timeout (1 sec)"=2000.0) -> ("error out"=w243:errorcluster, "watchdogID"=w244:u64)  [unwired: 1 in, 3 out]
            n120 = while {
              tunnel: [w267] -> w237
              tunnel: w244 -> [w315]
              tunnel: [w313] -> w241
              shift-right: [w251] -> w227
              shift-left: w233 -> [w269]
              shift-right: [w249] -> w225
              shift-left: w231 -> [w268]
              tunnel: w239 -> [w280]
              tunnel: w238 -> [w279]
              shift-right: [w278] -> w230
              shift-left: w243 -> [w314]
              i -> [w306]
              stop <- w317 stop-if-true
              # "Modificar F con\nfuente enchufada"
              # "Unir a detector de presencia,\nquitar fotocelula"
              # "El watchdog reinicia el sistema cuando las iteraciones tardan más de x segundo en este bucle"
              n121 = local read "Acelerómetros OK?"() -> (w277:bool[])
              n122 = local read "RFID_Error"() -> (w289:errorcluster)
              n123 = xnode "Read/Write Control"("FPGA VI Reference In"=w269, "error in"=w268) -> ("FPGA VI Reference Out"=w301:refnum<k20>, "error out"=w300:errorcluster, "DC OK"=w305:bool)
              n124 = Unbundle By Name(w289) -> ("status"=w287:bool)
              n125 = Index Array(array=w277, index #1=0 ("index"), index #2=1 ("index"), index #3=2 ("index"), index #4=3 ("index")) -> (element #1=→"Acel 1":bool, element #2=→"Acel 2":bool, element #3=→"Acel 3":bool, element #4=→"Acel 4":bool)
              n126 = call "ControlFuente.vi"("DC OK 3"=w305) -> ("DC OK 2"=→"Fuente":bool, "DC OK"=→"DC OK":string)  [unwired: 1 out]
              n127 = Not(x=w287) -> (.not. x?=→"RFID":bool)
              n128 = xnode "Read/Write Control"("FPGA VI Reference In"=w301, "error in"=w300) -> ("FPGA VI Reference Out"=w296:refnum<k20>, "error out"=w295:errorcluster, "Chassis Temperature"=w303:i16)
              n129 = call <vilib>:"RT LEDs.vi"("State"=1, "LED Num"=0) -> ()  [unwired: 1 in, 5 out]
              n130 = call "ControlFotocelula_V1.vi"("Tiempo de entrada a espera"=w280) -> ("Aviso no detección"=→"Aviso no detección":string, "Boolean"=w293:bool)
              "Fallo fotocelula" <- w293
              n131 = call "ControlTEST_V1.vi"("Días entre TEST 2"=i16 5, "Ultimo TEST"=w279, "Horario TEST"="05:59") -> ("Boolean"=w292:bool)  [unwired: 3 in]
              n132 = call <vilib>:"Watchdog Whack.vi"("error in (no error)"=w314, "reset watchdog after expire? (F)"=TRUE, "watchdogID in"=w315) -> ("error out"=w278:errorcluster, "watchdogID out"=w313:u64)  [unwired: 3 out]
              n133 = call "ControlTemperatura.vi"("Chassis Temperature"=w303) -> ("Aviso temperatura"=→"Aviso temperatura":string, "Boolean"=w297:bool, "T fuera rango"=→"T fuera rango":bool)
              n134 = xnode "Read/Write Control"("FPGA VI Reference In"=w296, "error in"=w295) -> ("FPGA VI Reference Out"=w272:refnum<k20>, "error out"=w271:errorcluster, "Detector de presencia"=w257:bool)
              n135 = Get Date/Time In Seconds() -> (seconds since 1Jan1904=w259:timestamp)
              n136 = Format Date/Time String(seconds (now)=w259, UTC format=FALSE) -> (date/time string=→"date/time string":string)  [unwired: 1 in]
              n137 = Compound Arithmetic op=OR(w297, FALSE ("value"), w293, w292) -> (w294:bool)
              n138 = case shown="True" "Adquirir continuado" {
                tunnel: ["Adquirir" TRUE ("Adquirir")] -> w266
                frame False {
                }
                frame True {
                  n139 = Wait (ms)(milliseconds to wait="milliseconds to wait") -> ()  [unwired: 1 out]
                }
              }
              n140 = call "Cambio_Fecha_Hora.vi"("Cambiar Fecha"="Cambiar Fecha", "Cambiar hora"="Cambiar hora", "Time"="Time", "Date"="Date") -> ()
              n141 = Compound Arithmetic op=OR("Parar la aplicación", "Reset del controlador", "Configuración", "Cambiar hora", "Cambiar Fecha") -> (w290:bool)
              n142 = xnode "Read/Write Control"("FPGA VI Reference In"=w272, "error in"=w271, "Fotocélula"=w266) -> ("FPGA VI Reference Out"=w252:refnum<k20>, "error out"=w250:errorcluster)
              n143 = Compound Arithmetic op=OR(w266, w294, w290, w257) -> (w317:bool)
              n144 = call "remove_files.vi"("Hora de borrado"="Hora de borrado") -> ()  [unwired: 1 in]
              n145 = Select(t="TEST", s=w294, f="Adquisición") -> (s? t:f=w309:string)
              n146 = xnode "Read/Write Control"("FPGA VI Reference In"=w252, "error in"=w250) -> ("FPGA VI Reference Out"=w251:refnum<k20>, "error out"=w249:errorcluster, "Direccion 0?"=→"Direccion 0?":bool)
              n147 = Select(t="Configuración", s=w290, f=w309) -> (s? t:f=w267:string)
              "Bucle Espera" <- w306
            }
            n148 = Unbundle By Name(w225) -> ("status"=w236:bool)
            n149 = Select(t="TEST", s=w236, f=w237) -> (s? t:f=w229:string)
            n150 = flat-sequence {
              tunnel: [w246] -> w228
              tunnel: w229 -> [w246]
              frame #0 {
                n151 = Get Date/Time In Seconds() -> (seconds since 1Jan1904=w247:timestamp)
                n152 = To Double Precision Float(number=w247) -> (double precision float=→"Tiempo":dbl)
              }
            }
            n153 = call <vilib>:"Watchdog Clear.vi"("error in (no error)"=w230, "watchdogID in"=w241) -> ("error out"=w226:errorcluster)  [unwired: 5 out]
          }
          frame "Adquisición" {
            n154 = local read "expiration actions"() -> (w326:T1)
            n155 = call <vilib>:"Watchdog Configure.vi"("error in (no error)"=w350, "expiration actions"=w326, "timeout (1 sec)"=200.0) -> ("error out"=w334:errorcluster, "watchdogID"=w335:u64)  [unwired: 3 out]
            n156 = flat-sequence {
              tunnel: w334 -> [w389]
              tunnel: w335 -> [w390]
              tunnel: w358 -> [w383]
              tunnel: w359 -> [w384]
              tunnel: [w390] -> w343
              tunnel: [w389] -> w342
              tunnel: [w382] -> w341
              tunnel: [w381] -> w340
              tunnel: [w380] -> w339
              tunnel: [w379] -> w338
              tunnel: [w378] -> w337
              tunnel: [w377] -> w336
              tunnel: [w360] -> w322
              tunnel: [w419] -> w356
              tunnel: [w403] -> w355
              tunnel: [w418] -> w354
              tunnel: [w417] -> w353
              tunnel: [w414] -> w352
              tunnel: [w407] -> w351
              tunnel: w343 -> [w416]
              tunnel: w342 -> [w415]
              tunnel: w341 -> [w413]
              tunnel: w340 -> [w412]
              tunnel: w339 -> [w411]
              tunnel: w338 -> [w410]
              tunnel: w337 -> [w409]
              tunnel: w336 -> [w408]
              tunnel: w323 -> [w406]
              tunnel: w322 -> [w401]
              tunnel: [w400] -> w321
              tunnel: w356 -> [w592]
              tunnel: w355 -> [w591]
              tunnel: w354 -> [w576]
              tunnel: w353 -> [w575]
              tunnel: w352 -> [w563]
              tunnel: [w599] -> w330
              tunnel: w351 -> [w602]
              tunnel: [w582] -> w345
              tunnel: [w583] -> w349
              tunnel: [w584] -> w348
              tunnel: [w592] -> w347
              tunnel: [w591] -> w346
              tunnel: w321 -> [w556]
              frame #0 {
                n157 = local read "Frecuencia de muestreo y módulo CRIO"() -> (w367:T5)
                n158 = local read "Count(mSec)"() -> (w364:u32)
                n159 = local read "Canal ccero?"() -> (w365:bool)
                n160 = local read "Offset_rueda"() -> (w363:fxp<+/-,24,-4>)
                n161 = local read "Digital?"() -> (w366:bool)
                n162 = xnode "Read/Write Control"("FPGA VI Reference In"=w384, "error in"=w383, "Data Rate"=w367, "Digital?"=w366, "Canal ccero?"=w365, "Count(mSec)"=w364, "Offset_rueda"=w363) -> ("FPGA VI Reference Out"=w373:refnum<k20>, "error out"=w372:errorcluster)
                n163 = local read "Frecuencia de muestreo (Hz)"() -> (w375:dbl)
                n164 = local read "RFID_LR6_Error"() -> (w361:errorcluster)
                n165 = call "DMACalc.vi"("Number of Channels"="Number of Channels", "Number of Samples"="Number of Samples", "Rate (Hz)"=w375) -> ("Block Size"=w379:u32, "Time to Acquire Block (ms)"=w380:i32, "Host Buffer Size"=w385:u32)  [unwired: 6 in]
                n166 = call "Pathhorafech(SubVI)_varios.vi"("Folder path"=path "c:/Trenes", "Nº de acelerómetros"=8, "Nº inductivos"=1) -> ("Acel_Paths"=w368:path[])  [unwired: 1 in, 1 out]
                "Nombre de archivo" <- w368
                n167 = call "LH6HD.vi"("error in (no error)"=w361, "Action"=enum16{"Init", "Start", "Read", "Stop", "Exit"}."Start") -> ("error out"=w360:errorcluster)  [unwired: 8 in, 1 out]
                n168 = for {
                  tunnel: w368 -> [w393] mode=indexing
                  tunnel: [w392] -> w378 mode=indexing
                  tunnel: [w391] -> w377
                  n169 = Open/Create/Replace File(file path (use dialog)=w393, operation (0:open)=T8."replace or create", access (0:read/write)=enum16{"read/write", "read-only", "write-only"}."read/write", disable buffering (F)=TRUE) -> (refnum out=w392:refnum<file>, error out=w391:errorcluster)  [unwired: 1 in, 2 out]
                }
                n170 = xnode "Invoke Method"("FPGA VI Reference In"=w373, "error in"=w372, "Requested Depth"=w385) -> ("FPGA VI Reference Out"=w388:refnum<k20>, "error out"=w387:errorcluster)  [unwired: 1 out]
                n171 = Get Date/Time In Seconds() -> (seconds since 1Jan1904=→"Inicio pasada":timestamp)
                n172 = xnode "Invoke Method"("FPGA VI Reference In"=w388, "error in"=w387) -> ("FPGA VI Reference Out"=w382:refnum<k20>, "error out"=w381:errorcluster)
              }
              frame #1 {
                n173 = while "Data Acquisition" {
                  tunnel: w413 -> [w460]
                  shift-right: [w489] -> _
                  shift-left: u32 0 ("t") -> [w485]
                  tunnel: w411 -> [w490]
                  tunnel: w410 -> [w488]
                  shift-right: [w491] -> w417
                  shift-left: w412 -> [w482]
                  tunnel: [w486] -> w418
                  tunnel: w409 -> [w466]
                  tunnel: [w467] -> w414
                  shift-right: [w465] -> w407
                  shift-left: w408 -> [w478]
                  tunnel: w406 -> [w462]
                  i -> [w459]
                  stop <- w487 stop-if-true
                  # "Detector de presencia"
                  # "Mide el tiempo de paso del tren y con ello se puede calcular\nla velocidad la unidad"
                  n174 = xnode "Invoke Method"("FPGA VI Reference In"=w460, "error in"=w482, "Number of Elements"=w485, "Timeout (ms)"=0) -> ("FPGA VI Reference Out"=w456:refnum<k20>, "error out"=w464:errorcluster, "Data"=w481:fxp<+/-,24,4>[], "Elements Remaining"=w483:u32)
                  n175 = case "Data Ready" shown="Default" w485 {
                    tunnel: w490 -> [w511 _]
                    tunnel: [w510 u32 0 ("t")] -> w489
                    tunnel: w488 -> [w512 _]
                    tunnel: w483 -> [w509 _]
                    tunnel: w481 -> [_ w533]
                    tunnel: w478 -> [w508 w532]
                    tunnel: [w508 w534] -> w465
                    tunnel: w466 -> [w507 w531]
                    tunnel: [w507 w530] -> w467
                    frame 0 {
                      # "En este caso se compara los elementos que quedan\nen la FIFO del controlador con el tamaño dell bloque\nque aparece en el panel frontal. Si el número de \nelementos en la FIFO es mayor o igual que el tamaño\n del bloque se pasa al siguiente caso y se guardan \nlos datos en un archivo. El reloj que aparece es una\nespera para no consumir recursos."
                      n176 = Greater Or Equal?(x=w509, y=w512) -> (x >= y?=w513:bool)
                      n177 = case shown="False" w513 {
                        tunnel: [u32 0 ("Block Size") w517] -> w510
                        tunnel: [w516 0 ("t")] -> w514
                        tunnel: w511 -> [w516 _]
                        tunnel: w512 -> [_ w517]
                        frame False {
                        }
                        frame True {
                        }
                      }
                      n178 = call "WaitMinTimeBetweenCall.vi"("Minimum ms between calls"=w514) -> ()  [unwired: 2 in]
                    }
                    frame Default {
                      n179 = To Single Precision Float(number=w533) -> (single precision float=w520:sgl[])
                      n180 = Decimate 1D Array(w520) -> (w526:sgl[], w529:sgl[], w528:sgl[], w527:sgl[], w525:sgl[], w524:sgl[], w523:sgl[], w522:sgl[], w521:sgl[])
                      n181 = Build Array(w526, w529, w528, w527, w525, w524, w523, w522, w521) -> (w519:sgl[][])
                      n182 = for {
                        tunnel: T9."little-endian" ("byte order (0:big-endian, network order)") -> [w543]
                        shift-right: [w537] -> w534
                        shift-left: w532 -> [w538]
                        tunnel: w519 -> [w541] mode=indexing
                        tunnel: w531 -> [w540] mode=indexing
                        tunnel: [w539] -> w530 mode=indexing
                        n183 = Write to Binary File(file (use dialog)=w540, data=w541, error in=w538, 5:FALSE ("prepend array or string size? (T)"), 9:w543) -> (refnum out=w539:refnum<file>, error out=w537:errorcluster)  [unwired: 2 out]
                      }
                    }
                  }
                  n184 = xnode "Read/Write Control"("FPGA VI Reference In"=w456, "error in"=w464) -> ("FPGA VI Reference Out"=w480:refnum<k20>, "error out"=w479:errorcluster, "Detector de presencia"=w472:bool)
                  n185 = case shown="True" w472 {
                    tunnel: [FALSE w502] -> w471
                    tunnel: [w493 w501] -> w470
                    tunnel: w462 -> [_ w498]
                    frame False {
                      n186 = local read "Inicio pasada"() -> (w496:timestamp)
                      n187 = Get Date/Time In Seconds() -> (seconds since 1Jan1904=w495:timestamp)
                      n188 = To Double Precision Float(number=w495) -> (double precision float=w492:dbl)
                      n189 = To Double Precision Float(number=w496) -> (double precision float=w497:dbl)
                      n190 = Subtract(x=w492, y=w497) -> (x-y=w493:dbl)
                      "Tiempo de paso (s)" <- w493
                      n191 = local write "Tiempo"(w492) -> ()
                    }
                    frame True {
                      (unwired) 0.0
                      n192 = local read "Tiempo extra al detector de paso (s)"() -> (w501:dbl)
                      n193 = local read "Tiempo"() -> (w506:dbl)
                      n194 = Get Date/Time In Seconds() -> (seconds since 1Jan1904=w503:timestamp)
                      n195 = To Double Precision Float(number=w503) -> (double precision float=w504:dbl)
                      n196 = Subtract(x=w504, y=w506) -> (x-y=w505:dbl)
                      "Tiempo extra de adquisición (s)" <- w505
                      n197 = Add(x="Tiempo de adquisicion", y=w498) -> (x+y=w499:dbl)
                      n198 = Greater?(x=w505, y=w499) -> (0:w502:bool)
                    }
                  }
                  "Fin" <- w471
                  n199 = xnode ("CheckLate")("FPGA VI Reference In"=w480, "error in"=w479) -> ("FPGA VI Reference Out"=w458:refnum<k20>, "error out"=w475:errorcluster, "Buffer Underflow"=→"Buffer Underflow":bool, "Buffer Overflow"=w461:bool)
                  "Buffer Overflow" <- w461
                  n200 = Greater?(x=w470, y=20.0) -> (0:w468:bool)
                  "Obstruido?" <- w468
                  n201 = call "ErrorOverFlow.vi"("Buffer Overflow"=w461) -> ("error out"=w473:errorcluster)
                  n202 = call "ErrorUnderFlow.vi"() -> ("error out"=w474:errorcluster)  [unwired: 1 in]
                  n203 = Merge Errors(w475, w474, w473) -> (w457:errorcluster)
                  n204 = Unbundle By Name(w465) -> ("status"=w469:bool)
                  n205 = Unbundle By Name(w457) -> ("status"=w477:bool)
                  n206 = Compound Arithmetic op=OR(w477, w471, w468, w469) -> (w487:bool)
                  "result" <- w487
                  n207 = case "Flush" shown="True" w487 {
                    tunnel: [w544 w549] -> w491
                    tunnel: [w545 w548] -> w486
                    tunnel: w458 -> [w545 w547]
                    tunnel: w457 -> [w544 w546]
                    frame False {
                    }
                    frame True {
                      n208 = xnode "Invoke Method"("FPGA VI Reference In"=w547, "error in"=w546) -> ("FPGA VI Reference Out"=w548:refnum<k20>, "error out"=w549:errorcluster)
                    }
                  }
                  "Block Size" <- w488
                  "Time to Acquire Block (ms)" <- w490
                  "Numeric 3" <- w459
                }
                n209 = call <vilib>:"Watchdog Whack.vi"("error in (no error)"=w415, "reset watchdog after expire? (F)"=TRUE, "watchdogID in"=w416) -> ("error out"=w404:errorcluster, "watchdogID out"=w419:u64)  [unwired: 3 out]
                n210 = while {
                  shift-right: [w427] -> w400
                  shift-left: w401 -> [w428]
                  shift-right: [w426] -> w399
                  shift-left: string[] [] -> [w425]
                  shift-right: [w421] -> w397
                  shift-left: i32[] [] -> [w422]
                  i -> [w423]
                  stop <- w424 stop-if-true
                  n211 = case shown="Error" w428 {
                    selector: w428 -> [w439 _]
                    tunnel: [w438 w453] -> w427
                    tunnel: [w434 string[] []] -> w426
                    tunnel: w425 -> [w433 _]
                    tunnel: w423 -> [w432 _]
                    tunnel: w422 -> [w431 _]
                    tunnel: [w430 i32[] []] -> w421
                    frame No Error {
                      n212 = call "LH6HD.vi"("error in (no error)"=w439, "Action"=enum16{"Init", "Start", "Read", "Stop", "Exit"}."Read") -> ("error out"=w438:errorcluster, "Tag"=w435:string)  [unwired: 8 in]
                      n213 = Not Equal?(x="", y=w435) -> (x != y?=w436:bool)
                      n214 = case shown="False" w436 {
                        tunnel: w435 -> [_ w448]
                        tunnel: [w442 w447] -> w434
                        tunnel: w433 -> [w442 w446]
                        tunnel: w432 -> [_ w443]
                        tunnel: w431 -> [w441 w445]
                        tunnel: [w441 w444] -> w430
                        frame False {
                        }
                        frame True {
                          n215 = Build Array (concatenate)(w446, w448) -> (w447:string[])
                          n216 = Build Array (concatenate)(w445, w443) -> (w444:i32[])
                        }
                      }
                    }
                    frame Error {
                      n217 = local read "LR6 IP address"() -> (w450:string)
                      n218 = local read "Port LR6"() -> (w451:u16)
                      n219 = call "LH6HD.vi"("DeviceAddress"=u8 0, "Reader Port"=w451, "IP Address"=w450, "Action"=enum16{"Init", "Start", "Read", "Stop", "Exit"}."Init") -> ("error out"=w453:errorcluster)  [unwired: 6 in, 1 out]
                    }
                  }
                  n220 = Wait Until Next ms Multiple(millisecond multiple=u32 500) -> ()  [unwired: 1 out]
                  n221 = local read "result"() -> (w424:bool)
                  "it-LR6" <- w423
                }
                "TAGs LR6" <- w399
                "it-read-LR6" <- w397
                n222 = Merge Errors(w404) -> (w403:errorcluster)
              }
              frame #2 {
                (unwired) u32 1000 ("Number of Elements")
                n223 = Array Size(array=w563) -> (size(s)=w561:i32)
                n224 = Decrement(x=w561) -> (x-1=w562:i32)
                n225 = local read "Puerto RFID"() -> (w581:u16)
                n226 = call "LH6HD.vi"("error in (no error)"=w556, "Action"=enum16{"Init", "Start", "Read", "Stop", "Exit"}."Stop") -> ("error out"=w555:errorcluster)  [unwired: 8 in, 1 out]
                n227 = local read "RFID_Error"() -> (w595:errorcluster)
                n228 = local read "IP RFID"() -> (w560:string)
                n229 = local read "RFID_ID"() -> (w594:refnum<k5>)
                n230 = Index Array(array=w563, index=w562) -> (element=w572:refnum<file>)
                n231 = local write "result"(FALSE ("result")) -> ()
                n232 = local write "RFID_LR6_Error"(w555) -> ()
                n233 = disable-structure shown="Enabled" {
                  disable-tunnel: [w626 _] -> w596
                  disable-tunnel: w595 -> [w625 w628]
                  disable-tunnel: w594 -> [w624 _]
                  disable-tunnel: [w623 _] -> w593
                  disable-tunnel: [w622 w628] -> w585
                  disable-tunnel: w581 -> [w621 _]
                  disable-tunnel: w560 -> [w620 _]
                  disable-tunnel: [w619 "TAGs HEX 2"] -> w553
                  frame Enabled {
                    n234 = call "RFID_28_03_12.vi"("RFID_Error"=w625, "Puerto RFID"=w621, "IP RFID"=w620, "RFID ID"=w624) -> ("Unidad"=w626:u32, "RFID Error"=w622:errorcluster, "connection ID out"=w623:refnum<k5>, "TAGs HEX"=w619:string[])  [unwired: 1 in]
                    "RFID_Error 2" <- w625
                  }
                  frame Disabled {
                  }
                }
                "TAGs HEX" <- w553
                n235 = local read "TAGs LR6"() -> (w554:string[])
                n236 = Index Array(array=w553) -> (element=w552:string)  [unwired: 1 in]
                n237 = Not Equal?(x=w552, y="" ("delimiter (\\t)")) -> (x != y?=w550:bool)
                "Plataformas?" <- w550
                n238 = case shown="True" w550 {
                  tunnel: w554 -> [w612 w613]
                  tunnel: [w612 w615] -> w558
                  tunnel: w553 -> [_ w614]
                  frame False {
                  }
                  frame True {
                    n239 = call "Union_TAGs_RFIDs.vi"("TAGs LR6"=w613, "TAGs HEX"=w614) -> ("TAGs"=w615:string[])
                  }
                }
                "TAGs" <- w558
                n240 = local read "Tiempo de paso (s)"() -> (w589:dbl)
                n241 = local read "Nombre de archivo"() -> (w571:path[])
                n242 = xnode "Read/Write Control"("FPGA VI Reference In"=w576, "error in"=w575) -> ("FPGA VI Reference Out"=w598:refnum<k20>, "error out"=w597:errorcluster, "Chassis Temperature"=w608:i16)
                n243 = Multiply(x=w589, y=1000.0) -> (x*y=w587:dbl)
                n244 = for {
                  shift-right: [w631] -> w579
                  shift-left: string[] [] -> [w630]
                  tunnel: w558 -> [w629] mode=indexing
                  n245 = Insert Into Array(array=w630, new element=w629) -> (w631:string[])  [unwired: 1 in]
                }
                n246 = Divide(x=w608, y=4.0) -> (x/y=w609:dbl)
                "Temperatura (ºC)" <- w609
                n247 = Build Array(w609, w587, w596) -> (w603:dbl[])
                n248 = local write "RFID_ID"(w593) -> ()
                n249 = local write "RFID_Error"(w585) -> ()
                n250 = Delete From Array(array=w571) -> (deleted portion=w570:path)  [unwired: 2 in, 1 out]
                n251 = To Single Precision Float(number=w603) -> (single precision float=w606:sgl[])
                n252 = xnode "Read/Write Control"("FPGA VI Reference In"=w598, "error in"=w597, "Stop"=TRUE ("stop")) -> ("FPGA VI Reference Out"=w574:refnum<k20>, "error out"=w573:errorcluster)
                n253 = Path To String(path=w570) -> (string=w578:string)
                n254 = Write to Binary File(file (use dialog)=w572, data=w606, error in=w602, 5:FALSE ("prepend array or string size? (T)"), 9:T9."little-endian" ("byte order (0:big-endian, network order)")) -> (error out=w569:errorcluster)  [unwired: 3 out]
                n255 = local read "Fin"() -> (w586:bool)
                n256 = Build Array (concatenate)(w578, w579) -> (w565:string[])
                n257 = local read "TAGS leidos"() -> (w564:path)
                n258 = local read "Obstruido?"() -> (w590:bool)
                n259 = for {
                  shift-right: [w618] -> w582
                  shift-left: w569 -> [w617]
                  tunnel: w563 -> [w616] mode=indexing
                  n260 = Close File(refnum=w616, error in=w617) -> (error out=w618:errorcluster)  [unwired: 1 out]
                }
                n261 = Select(t="Procesado", s=w586, f="Espera") -> (s? t:f=w601:string)
                n262 = xnode "Invoke Method"("FPGA VI Reference In"=w574, "error in"=w573) -> ("FPGA VI Reference Out"=w584:refnum<k20>, "error out"=w583:errorcluster)
                n263 = call-poly <vilib>:"Write To Spreadsheet File.vi"("delimiter (\\t)"=";" ("delimiter (\\t)"), "transpose? (no:F)"=FALSE, "append to file? (new file:F)"=TRUE, "1D data"=w565, "file path (dialog if empty)"=w564) -> ()  [unwired: 3 in, 1 out]
                n264 = Select(t="Escape", s=w590, f=w601) -> (s? t:f=w599:string)
              }
            }
            n265 = Random Number (0-1)() -> (number: 0 to 1=w325:dbl)
            n266 = Multiply(x=2, y=w325) -> (x*y=w323:dbl)
            n267 = call <vilib>:"Watchdog Clear.vi"("error in (no error)"=w346, "watchdogID in"=w347) -> ("error out"=w333:errorcluster)  [unwired: 5 out]
            n268 = Unbundle By Name(w349) -> ("status"=w331:bool)
            n269 = Unbundle By Name(w345) -> ("status"=w332:bool)
            n270 = Merge Errors(w345, w333) -> (w344:errorcluster)
            n271 = Compound Arithmetic op=OR(w331, w332) -> (w329:bool)
            n272 = Select(t="TEST", s=w329, f=w330) -> (s? t:f=w327:string)
          }
          frame "Procesado" {
            n273 = call <vilib>:"Watchdog Configure.vi"("error in (no error)"=w654, "expiration actions"="expiration actions", "timeout (1 sec)"=300.0) -> ("error out"=w652:errorcluster, "watchdogID"=w653:u64)  [unwired: 3 out]
            n274 = flat-sequence {
              tunnel: w653 -> [w666]
              tunnel: w652 -> [w665]
              tunnel: [w669] -> w636
              tunnel: [w664] -> w635
              tunnel: [w663] -> w634
              tunnel: [w845] -> w650
              tunnel: [w846] -> w651
              tunnel: [w847] -> w647
              tunnel: w636 -> [w847]
              tunnel: w635 -> [w846]
              tunnel: w634 -> [w845]
              frame #0 {
                n275 = flat-sequence {
                  tunnel: [w713] -> w668
                  tunnel: [w695] -> w667
                  tunnel: w666 -> [w720]
                  tunnel: w665 -> [w719]
                  tunnel: [w718] -> w664
                  tunnel: [w717] -> w663
                  tunnel: [w698] -> w662
                  tunnel: [w682] -> w661
                  tunnel: [w697] -> w660
                  tunnel: [w681] -> w659
                  frame #0 {
                    (unwired) string[] ["S200"] ("Series_flota1")
                    (unwired) i32[] [28] ("Ejes_UT")
                    (unwired) path "c:/0002_2010-05-08_08-07-07.bin" ("Nombre de archivo")
                    # "Unidad 514"
                    # "Señal del inductivo"
                    # "Estos indicadores sirven para controlar que no se sature la memoria"
                    # "Distancia de\nla unidad"
                    n276 = disable-structure shown="Enabled" {
                      disable-tunnel: [w722 string[] ["13690667", "6583", "6584"] ("Series_flota1")] -> w686
                      frame Disabled {
                        n277 = local read "TAGs"() -> (w722:string[])
                      }
                      frame Enabled {
                      }
                    }
                    n278 = disable-structure shown="Enabled" {
                      disable-tunnel: [w724 w726] -> w708
                      frame Disabled {
                        n279 = local read "Nombre de archivo"() -> (w724:path[])
                      }
                      frame Enabled {
                        n280 = Delete From Array(array="Array", index (col)="Índice de los archivos seleccionados") -> (deleted portion=w726:path[])  [unwired: 2 in, 1 out]
                      }
                    }
                    n281 = local read "Tabla_flota"() -> (w694:string[][])
                    n282 = call "Series_ejes_flota.vi"("Tabla_flota"=w694, "Tags"=w686) -> ("Nº Ejes"=w675:i32[], "Series del convoy"=w685:string[])  [unwired: 2 in, 1 out]
                    n283 = local read "Puntos medios de las ventanas"() -> (w696:dbl[][])
                    n284 = Array Size(array=w708) -> (size(s)=w705:i32)
                    n285 = Add Array Elements(numeric array=w675) -> (sum=w674:i32)
                    "Ejes_convoy" <- w674
                    n286 = Subtract(x=w705, y=1 ("length")) -> (x-y=w707:i32)
                    n287 = Array Size(array=w685) -> (size(s)=→"Nº UTs":i32)
                    n288 = Delete From Array(array=w708, index=w707) -> (deleted portion=w704:path, array with subset deleted=w697:path[])  [unwired: 1 in]
                    n289 = case shown="True" "Señal digital?" {
                      tunnel: [sgl[] [5.23] ("x*y") w731] -> _
                      frame False {
                      }
                      frame True {
                        n290 = Multiply(x=sgl 10.0, y="x*y") -> (x*y=w731:dbl[])
                      }
                    }
                    n291 = call <vilib>:"Watchdog Whack.vi"("error in (no error)"=w719, "reset watchdog after expire? (F)"=TRUE, "watchdogID in"=w720) -> ("error out"=w718:errorcluster, "watchdogID out"=w717:u64)  [unwired: 3 out]
                    n292 = Read from Binary File(5:sgl 0.0, 9:T9."little-endian" ("byte order (0:big-endian, network order)"), 10:-1 ("count (1)"), 11:w704) -> (0:w702:errorcluster, 2:w687:sgl[], 3:w703:refnum<file>)  [unwired: 1 in, 2 out]
                    n293 = Close File(refnum=w703, error in=w702) -> (error out=w698:errorcluster)  [unwired: 1 out]
                    n294 = local read "Series_flota"() -> (w693:string[])
                    n295 = call "Puntos medio de pulso.vi"("DI Inductivo"=w687) -> ("Puntos"=w713:sgl[], "Número de ejes"=w672:i32)  [unwired: 1 in]
                    n296 = Array Size(array=w687) -> (size(s)=w692:i32)
                    n297 = call "Distancias_ejes_convoy.vi"("Series_flota1"=w685, "Ejes_UT"=w675, "Puntos medios de las ventanas"=w696, "Series_flota"=w693) -> ("Distancias_entre_ejes_convoy"=w695:dbl[])  [unwired: 1 in]
                    n298 = Subtract(x=w692, y=3 ("length")) -> (x-y=w690:i32)
                    n299 = Delete From Array(array=w687, length=3, index=w690) -> (array with subset deleted=w688:sgl[])  [unwired: 1 out]
                    n300 = Decrement(x=w672) -> (x-1=w712:i32)
                    n301 = local read "Tiempo de paso (s)"() -> (w711:dbl)
                    n302 = local read "TAGs"() -> (w680:string[])
                    n303 = local read "it-LR6"() -> (w677:i32)
                    n304 = local read "it-read-LR6"() -> (w678:i32[])
                    n305 = local read "TAGs LR6"() -> (w679:string[])
                    n306 = local read "Plataformas?"() -> (w676:bool)
                    n307 = call "Calculo_Velocidad.vi"("Tiempo de paso (s)"=w711, "Ejes"=w712, "Puntos iniciales de las ventanas"=w695) -> ("V (m/s)"=→"V (m/s)":dbl, "Longitud de la unidad"=→"Longitud de la unidad":dbl)
                    n308 = call "TAGs_AURAwheel.vi"("Nº Ejes"=w675, "TAGs"=w680, "Ejes_convoy"=w674, "it-LR6"=w677, "TAGs LR6"=w679, "it-read-LR6"=w678, "Plataformas?"=w676) -> ("TAGS_AURA"=→"TAGs_AURAwheel":string[][])  [unwired: 1 in]
                    n309 = call "Comprobación Señal digital (SubVI).vi"("Inductivo"=w688) -> ("Señal digital?"=w683:bool)
                    n310 = Get Volume Info(11:path "c:/" ("path")) -> (1:→"Disco Duro Disponible (bytes)":i64)  [unwired: 1 in, 5 out]
                    n311 = Equal?(x=w672, y=w672) -> (x = y?=w681:bool)
                    n312 = And(x=w681, y=w683) -> (x .and. y?=w682:bool)
                    "Número de ejes detectados" <- 3 ("Número de ejes detectados")
                    "Nº Ejes" <- i32[] [3, 3] ("Nº Ejes")
                  }
                }
                n313 = case shown="True" w661 {
                  tunnel: w662 -> [w734 w764]
                  tunnel: [w734 w763] -> w669
                  tunnel: w668 -> [_ w768]
                  tunnel: w667 -> [_ w766]
                  tunnel: w660 -> [_ w767]
                  tunnel: w659 -> [w732 _]
                  frame False {
                    n314 = local read "Nombre de archivo"() -> (w733:path[])
                    n315 = for {
                      tunnel: w733 -> [w736] mode=indexing
                      tunnel: w732 -> [w735]
                      n316 = flat-sequence {
                        tunnel: w736 -> [w745]
                        tunnel: [w745] -> w739
                        tunnel: [w744] -> w738
                        tunnel: w735 -> [w743]
                        tunnel: w739 -> [w752]
                        tunnel: [w751] -> w737
                        tunnel: w738 -> [w751]
                        tunnel: w737 -> [w754]
                        frame #0 {
                          w744 = path "c:/Est_Adq.csv" ("file path (use dialog)")
                          n317 = Path To String(path=w745) -> (string=w747:string)
                          n318 = Select(t="Nº Ejes detectados WS diferente a Nº Ejes TAGs" ("delimiter (\\t)"), s=w743, f="La señal del inductivo no es digital" ("delimiter (\\t)")) -> (s? t:f=w740:string)
                          n319 = Build Array(w747, w740) -> (w746:string[])
                          n320 = call-poly <vilib>:"Write To Spreadsheet File.vi"("delimiter (\\t)"=";" ("delimiter (\\t)"), "transpose? (no:F)"=FALSE, "append to file? (new file:F)"=TRUE, "1D data"=w746, "file path (dialog if empty)"=w744) -> ()  [unwired: 3 in, 1 out]
                        }
                        frame #1 {
                          n321 = disable-structure shown="Disabled" {
                            disable-tunnel: w752 -> [w753 _]
                            frame Disabled {
                              n322 = Delete(path (use dialog)=w753) -> ()  [unwired: 1 in, 6 out]
                            }
                            frame Enabled {
                            }
                          }
                        }
                        frame #2 {
                          n323 = File/Directory Info(path=w754) -> (size=w757:i64)  [unwired: 1 in, 6 out]
                          n324 = Greater?(x=w757, y=i64 1000000) -> (0:w755:bool)
                          n325 = case shown="True" w755 {
                            tunnel: w754 -> [_ w758]
                            frame False {
                            }
                            frame True {
                              n326 = Delete(path (use dialog)=w758) -> ()  [unwired: 4 in, 3 out]
                            }
                          }
                        }
                      }
                    }
                  }
                  frame True {
                    n327 = flat-sequence {
                      tunnel: w768 -> [w835]
                      tunnel: w767 -> [w831]
                      tunnel: w766 -> [w836]
                      tunnel: [w829] -> w765
                      frame #0 {
                        # "Entrada:\n- dt RMS\n- Paths\n- Param_acelerometros (sensivity)\n- Parm_filtro\n- Puntos ventana\n- error\n- Frecuencia\n- Velocidad ejes\n- Punto medio paso rueda (p)"
                        # "SALIDA \n\nMáximos por rueda inductivo"
                        # "ENTRADA \nNúmero de ejes\nDistancia de acelerómetros\nDistancias del centro de las ruedas\nPuntos medios de las ruedas (INDUCTIVO)\nFrecuencia\ndt RMS\nDistancias generales\nAceleraciones"
                        # "8 acelerómetros"
                        # "Velocidad"
                        n328 = local read "Frecuencia de muestreo (Hz)"() -> (w834:dbl)
                        n329 = local read "Direccion 0?"() -> (w826:bool)
                        n330 = local read "Distancia de acelerómetros"() -> (w837:dbl[])
                        n331 = local read "Parámetros acelerómetros"() -> (w828:dbl[])
                        n332 = local read "Número de ejes detectados"() -> (w827:i32)
                        n333 = local read "Distancias generales"() -> (w832:dbl[])
                        n334 = local read "dt RMS"() -> (w833:dbl)
                        n335 = call "Procesado_aRMS_BIdirecc.vi"("Paths_canales_aRMS"=w831, "Distancias generales (m)"=w832, "Distancias\nacelerometros"=w837, "Ejes Procesados"=w827, 5:w826, "Distancias centrales de las ruedas\n               configuración (m)"=w836, "Frecuencia de muestreo"=w834, "Parámetros acelerómetros"=w828, "dt RMS 2"=w833, "Puntos"=w835) -> ("Max RMS Ruedas"=w830:dbl[][])
                        n336 = Transpose 2D Array(2D array=w830) -> (transposed array=w829:dbl[][])
                        "Max RMS Ruedas" <- w829
                      }
                    }
                    n337 = disable-structure shown="Disabled" {
                      disable-tunnel: [w824 TRUE ("Use Aura?")] -> w762
                      frame Disabled {
                        n338 = local read "Use Aura?"() -> (w824:bool)
                      }
                      frame Enabled {
                      }
                    }
                    n339 = local read "TAGs_AURAwheel"() -> (w760:string[][])
                    n340 = local read "Nº Ejes"() -> (w759:i32[])
                    n341 = for {
                      tunnel: w762 -> [w773]
                      tunnel: [w772] -> w761 mode=indexing
                      tunnel: w760 -> [w771] mode=indexing
                      shift-right: [w770] -> _
                      shift-left: w765 -> [w774]
                      tunnel: w759 -> [w769] mode=indexing
                      # "dev.api.aurawheel.com"
                      n342 = case shown="True" w773 {
                        tunnel: w774 -> [w775 w781]
                        tunnel: [errorcluster {"status"=FALSE, "code"=0, "source"=""} ("error out") w793] -> w772
                        tunnel: w771 -> [_ w782]
                        tunnel: [w775 w780] -> w770
                        tunnel: w769 -> [_ w778]
                        frame False {
                        }
                        frame True {
                          (unwired) "http://dev.api.aurawheel.com/services/wrd/upload"
                          (unwired) "tagMexFin"
                          (unwired) "tagMexInit"
                          (unwired) "tag2"
                          (unwired) "tag1"
                          w797 = cluster{"status":string} {"status"=""}
                          n343 = local read "TAGs"() -> (w788:string[])
                          n344 = local read "Parametros AuraWheel"() -> (w822:string[])
                          n345 = Delete From Array(array=w781, length=w778, index (row)=0) -> (deleted portion=w777:dbl[][], array with subset deleted=w780:dbl[][])  [unwired: 1 in]
                          n346 = Get Date/Time In Seconds() -> (seconds since 1Jan1904=w818:timestamp)
                          n347 = Delete From Array(array=w788, length=2, index=0) -> ()  [unwired: 2 out]
                          n348 = Format Date/Time String(time format string (%c)="%H:%M:%S%3u", seconds (now)=w818) -> (date/time string=w816:string)  [unwired: 1 in]
                          n349 = Get Date/Time In Seconds() -> (seconds since 1Jan1904=w792:timestamp)
                          n350 = Scan From String(format string="%d:%d:%f", input string=w816) -> (output 1=w813:i32, output 2=w812:i32, output 3=w810:dbl)  [unwired: 5 in, 3 out]
                          n351 = local read "Temperatura (ºC)"() -> (w790:dbl)
                          n352 = disable-structure shown="Enabled" {
                            disable-tunnel: [_ 60.0 ("p_sp")] -> w789
                            frame Disabled {
                              n353 = local read "V (m/s)"() -> ()  [unwired: 1 out]
                            }
                            frame Enabled {
                            }
                          }
                          n354 = Multiply(x=w810, y=1000.0) -> (x*y=w806:dbl)
                          n355 = call "Time_to_ms.vi"("seconds since 1Jan1904"=w792) -> ("Numeric"=w791:dbl)  [unwired: 1 in]
                          n356 = Multiply(x=w812, y=60000) -> (x*y=w807:i32)
                          n357 = Multiply(x=3600000, y=w813) -> (x*y=w808:i32)
                          n358 = Index Array(array=w822) -> ()  [unwired: 3 in, 3 out]
                          n359 = call "aw_WRDCluster_8acel.vi"("Array TAGs"=w782, "Max RMS Ruedas"=w777, "TimeStamp"=w791, "p_sp"=w789, "p_tp"=w790) -> ("JSON cluster"=w819:T11)  [unwired: 1 in]
                          n360 = Compound Arithmetic op=ADD(w808, w807, w806) -> (w805:dbl)
                          n361 = To Variant(anything=w819) -> (Variant=w802:variant)
                          n362 = To Unsigned Long Integer(number=w805) -> (unsigned 32bit integer=w804:u32)
                          n363 = call "gjson_Create.vi"("JSON Object in"=w802) -> ("error out"=w800:errorcluster, "JSON String Out"=w801:string)  [unwired: 9 in]
                          n364 = Number To Decimal String(number=w804) -> (decimal integer string=w803:string)  [unwired: 1 in]
                          n365 = To Variant(anything=w797) -> (Variant=w796:variant)
                          n366 = call "aw_SendData.vi"("pwd"="wrd", "x-nem-datetime"=w803, "User"="User", "error in"=w800, "JSON Object"=w801, "URL"="http://api.aurawheel.dev/services/wrd/upload") -> ("error out"=w798:errorcluster, "Response JSON"=w799:string, "Response headers"=→"Response headers":string)  [unwired: 3 in]
                          n367 = call "gjson_Parse.vi"("error in"=w798, "JSON String In"=w799, "JSON Cluster"=w796) -> ("error out"=w794:errorcluster, "JSON Cluster Out"=w795:variant)  [unwired: 7 in]
                          n368 = Variant To Data(error in=w794, type=w797, Variant=w795) -> (data=→"data":cluster{"status":string}, error out=w793:errorcluster)
                          "error AURA" <- w793
                        }
                      }
                    }
                    n369 = Merge Errors(w761, w764) -> (w763:errorcluster)
                  }
                }
              }
              frame #1 {
                n370 = local read "TAGS leidos"() -> (w841:path)
                n371 = local read "Nombre de archivo"() -> (w838:path[])
                n372 = File/Directory Info(path=w841) -> (size=w844:i64)  [unwired: 1 in, 6 out]
                n373 = local read "Path TEST"() -> (w840:path)
                n374 = disable-structure shown="Disabled" {
                  frame Disabled {
                    n375 = call "Borrar_carpeta.vi"("Nº Archivos Max"=1000, "Path Carpeta"=path "c:/Trenes") -> ()  [unwired: 1 in]
                  }
                  frame Enabled {
                  }
                }
                n376 = Greater?(x=w844, y=i64 1000000) -> (0:w842:bool)
                n377 = case shown="True" w842 {
                  tunnel: w841 -> [_ w850]
                  frame False {
                  }
                  frame True {
                    n378 = Delete(path (use dialog)=w850) -> ()  [unwired: 4 in, 3 out]
                  }
                }
                n379 = call "Borrar_carpeta.vi"("Nº Archivos Max"=i64 250 ("y"), "Path Carpeta"=w840) -> ()  [unwired: 1 in]
                n380 = call "Retrieve_memory_3_folders.vi"() -> ()  [unwired: 12 in]
                n381 = call "Comprimir_a_1_archivo.vi"("Acel_paths"=w838) -> ()  [unwired: 1 out]
              }
            }
            n382 = disable-structure shown="Disabled" {
              disable-tunnel: [w658 _] -> w632
              frame Disabled {
                n383 = local read "IP synchr"() -> (w657:string)
                n384 = call "Synchronization.vi"("Time Server\nIP Address"=w657) -> ("error out"=w658:errorcluster)
              }
              frame Enabled {
              }
            }
            n385 = call <vilib>:"Watchdog Clear.vi"("error in (no error)"=w651, "watchdogID in"=w650) -> ("error out"=w649:errorcluster)  [unwired: 5 out]
            n386 = local read "RFID_Error"() -> (w637:errorcluster)
            n387 = Merge Errors(w647, w649) -> (w638:errorcluster)
            n388 = Merge Errors(w633, w632, w637, w638) -> (w648:errorcluster)
            n389 = Unbundle By Name(w648) -> ("status"=w642:bool)
            n390 = Select(t="Descarga datos", s=FALSE, f="Espera") -> (s? t:f=w644:string)
            n391 = Select(t="TEST", s=w642, f=w644) -> (s? t:f=w641:string)
          }
          frame "TEST" {
            n392 = local read "expiration actions"() -> (w852:T1)
            n393 = call <vilib>:"Watchdog Configure.vi"("expiration actions"=w852, "timeout (1 sec)"=200.0) -> ("error out"=w855:errorcluster, "watchdogID"=w856:u64)  [unwired: 1 in, 3 out]
            n394 = flat-sequence {
              tunnel: [w867] -> w862
              tunnel: w861 -> [w887]
              tunnel: w859 -> [w886]
              tunnel: [w885] -> w858
              tunnel: w856 -> [w876]
              tunnel: w855 -> [w875]
              tunnel: [w874] -> w854
              tunnel: [w873] -> w853
              tunnel: [w863] -> w851
              frame #0 {
                n395 = call <vilib>:"Watchdog Whack.vi"("error in (no error)"=w875, "reset watchdog after expire? (F)"=TRUE, "watchdogID in"=w876) -> ("error out"=w873:errorcluster, "watchdogID out"=w874:u64)  [unwired: 3 out]
                n396 = Get Date/Time In Seconds() -> (seconds since 1Jan1904=w879:timestamp)
                n397 = local read "Ultimo TEST"() -> (w880:timestamp)
                n398 = To Double Precision Float(number=w879) -> (double precision float=w881:dbl)
                n399 = Subtract(x=w881, y=3600.0) -> (x-y=w883:dbl)
                n400 = To Time Stamp(1:w883) -> (0:w884:timestamp)
                n401 = In Range and Coerce(upper limit=w879, x=w880, lower limit=w884) -> (In Range?=w878:bool)  [unwired: 1 out]
                n402 = case shown="False" w878 {
                  tunnel: w887 -> [w917 _]
                  tunnel: w886 -> [w892 w923]
                  tunnel: [w902 errorcluster {"status"=FALSE, "code"=0, "source"=""} ("error out")] -> w885
                  tunnel: [w892 w923] -> w863
                  frame False {
                    n403 = local read "Obstruido?"() -> (w894:bool)
                    n404 = case shown="True" w894 {
                      selector: w894 -> [_ w919]
                      tunnel: ["\r" w920] -> w891
                      frame False {
                      }
                      frame True {
                        n405 = call "ErrorObstruccion.vi"("Buffer Overflow"=w919) -> ("error out"=w922:errorcluster)
                        n406 = call "Error.vi"("Error con..."="Warning:", "error comunicacion 2"=w922) -> ("String"=w920:string)
                      }
                    }
                    n407 = local read "Aviso no detección"() -> (w900:string)
                    n408 = local read "Aviso temperatura"() -> (w899:string)
                    n409 = local read "RFID_Error"() -> (w896:errorcluster)
                    n410 = local read "RFID_LR6_Error"() -> (w889:errorcluster)
                    n411 = local read "DC OK"() -> (w898:string)
                    n412 = local read "Fallo sensores"() -> (w893:string)
                    n413 = call "Cabecera.vi"() -> ("String"=w915:string)
                    n414 = call "Adquisicion.vi"("Aviso no detección"=w900) -> ("String"=w914:string)
                    n415 = call "Temperatura.vi"("Aviso temperatura"=w899) -> ("String"=w913:string)
                    n416 = call "Fuente.vi"("DC OK"=w898) -> ("String"=w912:string)
                    n417 = call "FPGA.vi"("error out"=w892) -> ("String"=w911:string)
                    n418 = call "Escritura.vi"("error out"=w917) -> ("String"=w910:string)
                    n419 = call "Error.vi"("Error con..."="Error con el lecto RFID NEM", "error comunicacion 2"=w896) -> ("String"=w895:string)
                    n420 = call "Error.vi"("Error con..."="Error con el lecto RFID LR6-HD", "error comunicacion 2"=w889) -> ("String"=w888:string)
                    n421 = Concatenate Strings(w915, w914, w913, w912, w911, w910, w893, w895, w888, w891) -> (w916:string)
                    n422 = call "STRINGhorafechA(SubVI).vi"() -> ("STRINGhora_fecha"=w909:string)
                    n423 = Concatenate Strings(w909, ".txt" ("string")) -> (w905:string)
                    n424 = Get Date/Time In Seconds() -> (seconds since 1Jan1904=→"Ultimo TEST":timestamp)
                    n425 = Build Array("c", "TEST" ("element"), w905) -> (w907:string[])
                    n426 = Array of Strings to Path(0:w907) -> (2:w903:path)  [unwired: 1 out]
                    n427 = Write to Text File(file (use dialog)=w903, text=w916) -> (error out=w902:errorcluster)  [unwired: 1 in, 3 out]
                  }
                  frame True {
                  }
                }
                n428 = local read "Fallo fotocelula"() -> (w866:bool)
                n429 = Unbundle By Name(w863) -> ("status"=w864:bool)
                n430 = local read "T fuera rango"() -> (w872:bool)
                n431 = Compound Arithmetic op=OR(w864, w866) -> (w865:bool)
                n432 = local write "Reset del controlador"(w865) -> ()
                n433 = Select(t="Escape", s=w872, f="Espera") -> (s? t:f=w869:string)
                n434 = Select(t="Configuracion", s=w865, f=w869) -> (s? t:f=w867:string)
              }
            }
            n435 = call <vilib>:"Watchdog Clear.vi"("error in (no error)"=w853, "watchdogID in"=w854) -> ()  [unwired: 6 out]
          }
          frame "Escape" {
            n436 = while {
              tunnel: w928 -> [w944]
              tunnel: [w943] -> w929
              shift-right: [w942] -> w926
              shift-left: w925 -> [w931]
              stop <- w934 stop-if-true
              # "Espera hasta que el detector de\npresencia se desactive"
              n437 = Wait (ms)(milliseconds to wait=u32 3000) -> ()  [unwired: 1 out]
              n438 = xnode "Read/Write Control"("FPGA VI Reference In"=w944, "error in"=w931) -> ("FPGA VI Reference Out"=w943:refnum<k20>, "error out"=w942:errorcluster, "Detector de presencia"=w940:bool, "Chassis Temperature"=w935:i16)
              n439 = Divide(x=w935, y=4.0) -> (x/y=w936:dbl)
              n440 = In Range and Coerce(upper limit=55.0, x=w936, lower limit=0.0) -> (In Range?=w932:bool)  [unwired: 1 out]
              n441 = Not(x=w940) -> (.not. x?=w933:bool)
              n442 = And(x=w933, y=w932) -> (x .and. y?=w934:bool)
            }
          }
        }
        "Estado" <- w66
        "error manipulacion archivos" <- w68
        n443 = local read "Parar la aplicación"() -> (w65:bool)
      }
      n444 = xnode "Close FPGA VI Reference"("FPGA VI Reference In"=w58, "error in"=w57) -> ("error out"=→"error FPGA":errorcluster)
    }
    frame #3 {
      n445 = local read "RFID_ID"() -> (w947:refnum<k5>)
      n446 = call "LH6HD.vi"("Action"=enum16{"Init", "Start", "Read", "Stop", "Exit"}."Stop") -> ("error out"=→"RFID_LR6_Error":errorcluster)  [unwired: 9 in, 1 out]
      n447 = TCP Close Connection(connection ID=w947) -> (error out=→"RFID_Error":errorcluster)  [unwired: 1 in, 2 out]
    }
  }
